vi "Write SerDes GPIO Bank.vi"(0 "gpio bank output":T2, 2 "serdes id":T1=enum."SI 0 Deserializer") -> (4 "serdes id valid":bool)   [LabVIEW 2020, in "GettingStarted_Common_148X_FPGA.lvlib"]
uses:
  GettingStarted_Common_148X_FPGA.lvlib
  <instrlib>/FlexRIO/CSI-2/v2/FPGA/Types/GPIO Bank.ctl
  Types/SerDes Identifier.ctl
  <instrlib>/_niInstr/Basic Elements/v1/FPGA/niInstr Basic Elements v1 FPGA.lvlib
  <vilib>/eio/EIONode/EIONode.xnode
  <vilib>/rvi/eio/common/nirviEmuTemplateMethod_errors.vi
  <instrlib>/FlexRIO/CSI-2/v2/FPGA/NI CSI-2 API FPGA v2.lvlib
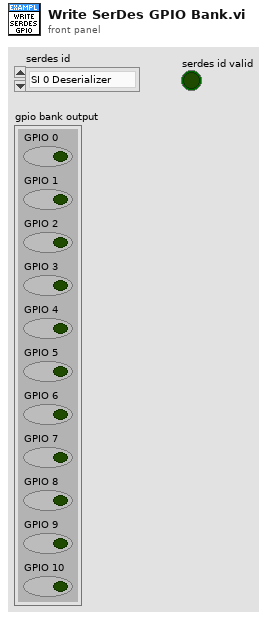
[diagram p1: front panel]
types:
  T1 = typedef "GettingStarted_Common_148X_FPGA.lvlib/SerDes Identifier.ctl" = enum8{"None", "SI 0 Deserializer", "SI 1 Deserializer", "SI 2 Deserializer", "SI 3 Deserializer", "SI 4 Deserializer", "SI 5 Deserializer", "SI 6 Deserializer", "SI 7 Deserializer", "SO 0 Serializer", "SO 1 Serializer", "SO 2 Serializer", "SO 3 Serializer", "SO 4 Serializer", "SO 5 Serializer", "SO 6 Serializer", "SO 7 Serializer", "SI 0 SI 1 Deserializer", "SI 2 SI 3 Deserializer", "SI 4 SI 5 Deserializer", "SI 6 SI 7 Deserializer"}
  T2 = typedef "NI CSI-2 API FPGA v2.lvlib/GPIO Bank.ctl" = cluster{"GPIO 0":bool, "GPIO 1":bool, "GPIO 2":bool, "GPIO 3":bool, "GPIO 4":bool, "GPIO 5":bool, "GPIO 6":bool, "GPIO 7":bool, "GPIO 8":bool, "GPIO 9":bool, "GPIO 10":bool}
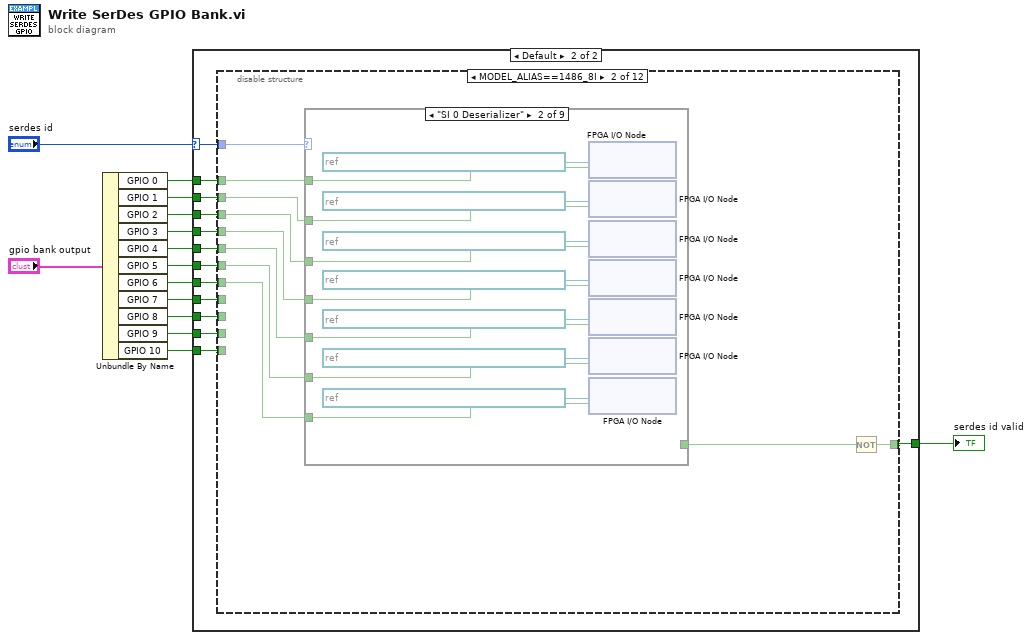
[diagram p0: block diagram]
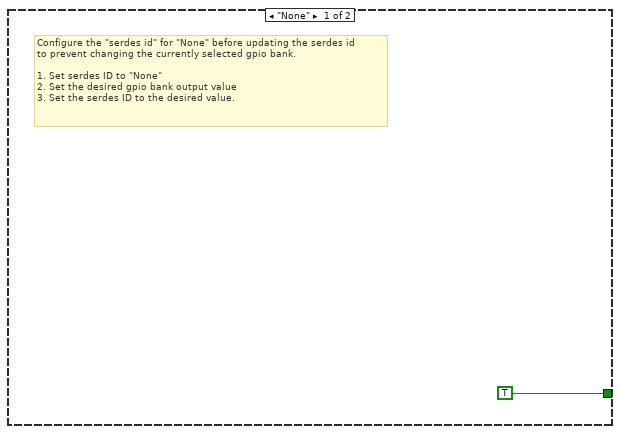
[diagram p2: hidden frame]
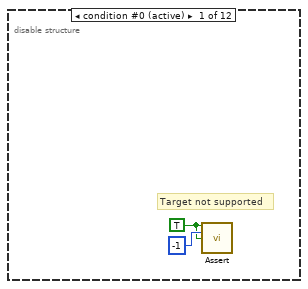
[diagram p3: hidden frame]
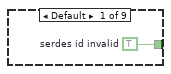
[diagram p4: hidden frame]
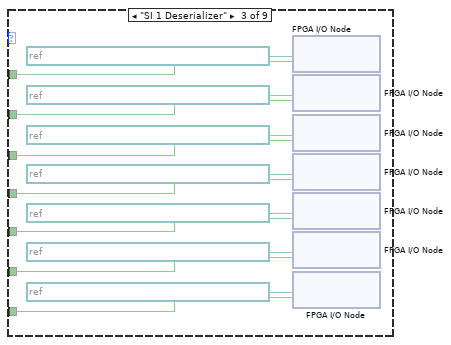
[diagram p5: hidden frame]
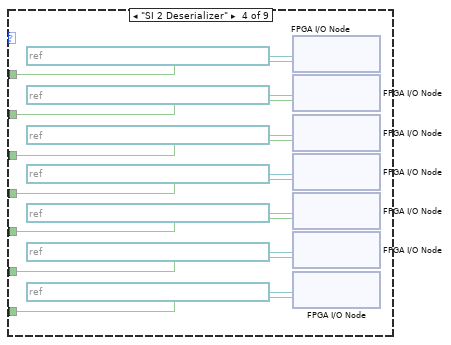
[diagram p6: hidden frame]
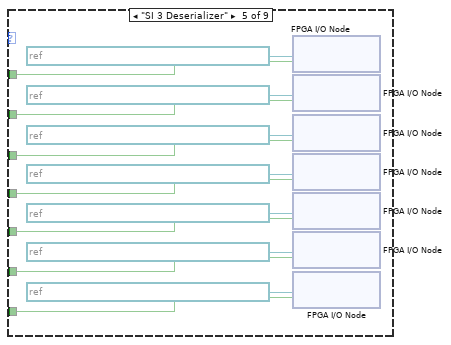
[diagram p7: hidden frame]
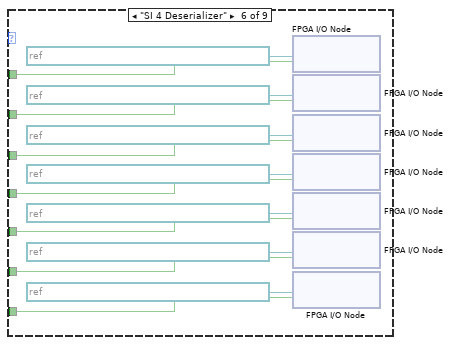
[diagram p8: hidden frame]
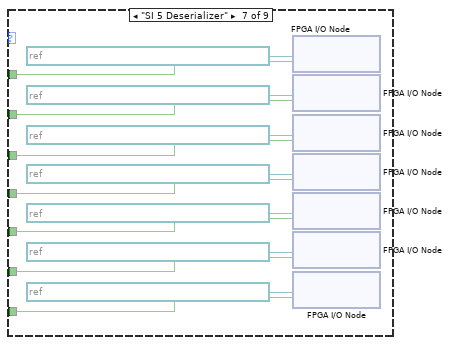
[diagram p9: hidden frame]
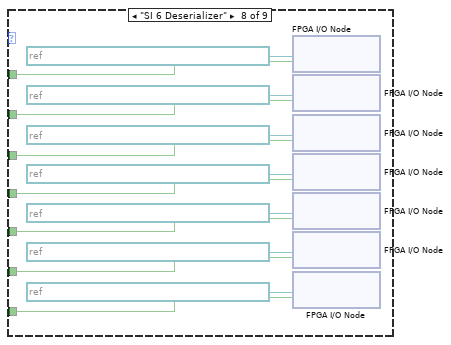
[diagram p10: hidden frame]
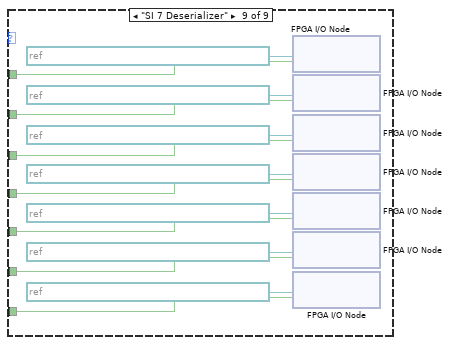
[diagram p11: hidden frame]
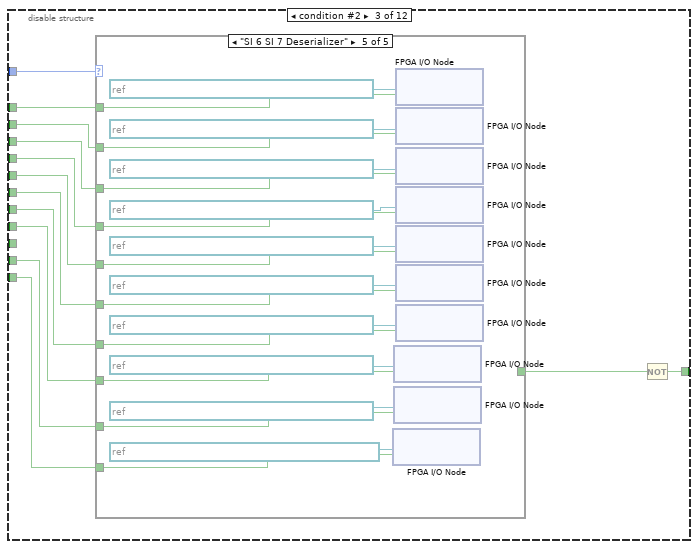
[diagram p12: hidden frame]
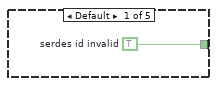
[diagram p13: hidden frame]
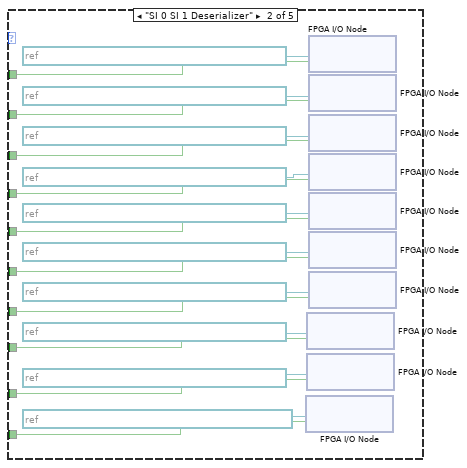
[diagram p14: hidden frame]
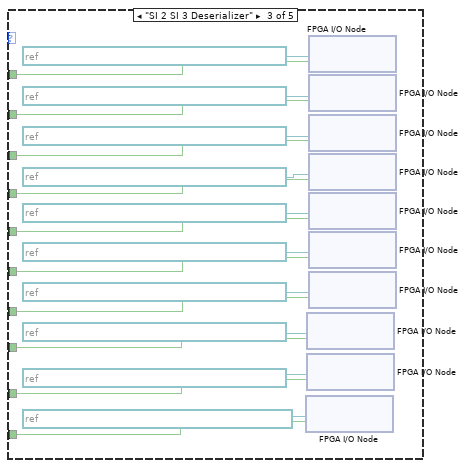
[diagram p15: hidden frame]
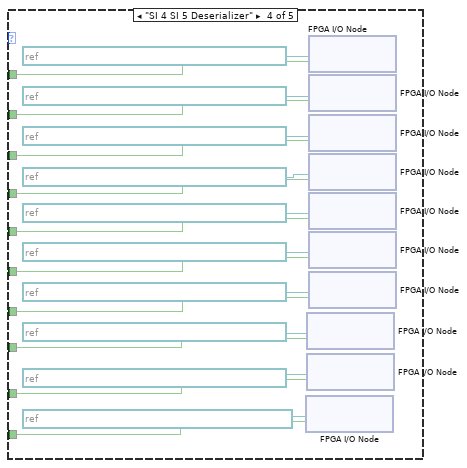
[diagram p16: hidden frame]
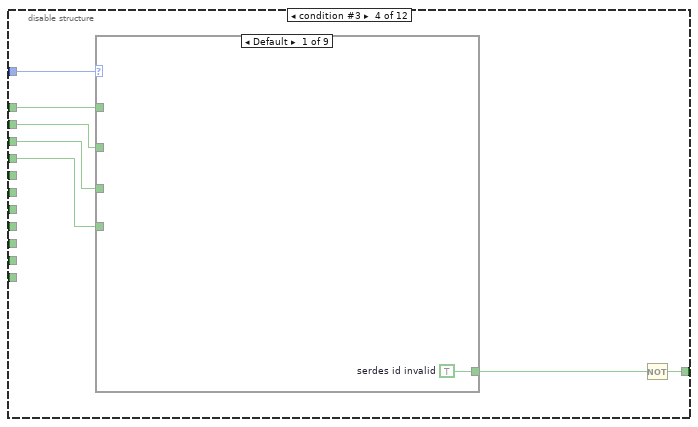
[diagram p17: hidden frame]
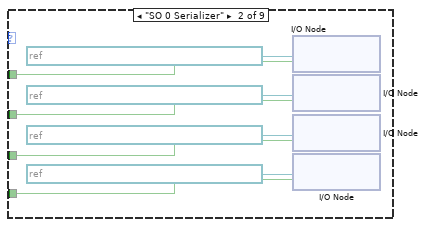
[diagram p18: hidden frame]
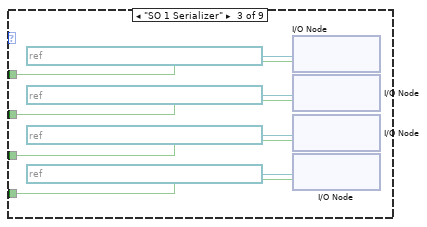
[diagram p19: hidden frame]
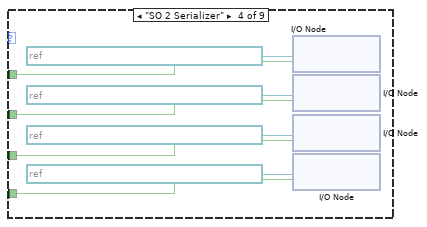
[diagram p20: hidden frame]
diagram:
  n1 = Unbundle By Name("gpio bank output") -> ("GPIO 0"=w13:bool, "GPIO 1"=w12:bool, "GPIO 2"=w11:bool, "GPIO 3"=w10:bool, "GPIO 4"=w9:bool, "GPIO 5"=w8:bool, "GPIO 6"=w7:bool, "GPIO 7"=w6:bool, "GPIO 8"=w5:bool, "GPIO 9"=w4:bool, "GPIO 10"=w3:bool)
  n2 = case shown="Default" "serdes id" {
    selector: "serdes id" -> [_ w16]
    tunnel: w13 -> [_ w28]
    tunnel: w12 -> [_ w27]
    tunnel: w11 -> [_ w26]
    tunnel: w10 -> [_ w25]
    tunnel: w9 -> [_ w24]
    tunnel: w8 -> [_ w23]
    tunnel: w7 -> [_ w22]
    tunnel: w6 -> [_ w21]
    tunnel: w5 -> [_ w20]
    tunnel: w4 -> [_ w19]
    tunnel: w3 -> [_ w18]
    tunnel: [TRUE w17] -> w2
    frame "None" {
      # "Configure the \"serdes id\" for \"None\" before updating the serdes id\nto prevent changing the currently selected gpio bank.\n\n1. Set serdes ID to \"None\" \n2. Set the desired gpio bank output value \n3. Set the serdes ID to the desired value."
    }
    frame Default {
      n3 = disable-structure shown="MODEL_ALIAS==1486_8I" {
        disable-tunnel: w16 -> [_ w40 w166 w254 w329 w431 w558 w645 w691 w797 w860 w995]
        disable-tunnel: w28 -> [_ w39 w165 w253 w328 w430 w557 w644 w690 w796 w859 w994]
        disable-tunnel: w27 -> [_ w38 w164 w252 w327 w429 w556 w643 _ _ w858 w993]
        disable-tunnel: w26 -> [_ w37 w163 w251 w326 w428 w555 w642 _ _ w857 w992]
        disable-tunnel: w25 -> [_ w36 w162 w250 w325 w427 w554 w641 w689 w795 w856 w991]
        disable-tunnel: w24 -> [_ w35 w161 _ w324 w426 w553 w640 w688 w794 w855 w990]
        disable-tunnel: w23 -> [_ w34 w160 _ w323 w425 w552 w639 _ _ w854 w989]
        disable-tunnel: w22 -> [_ w33 w159 _ w322 w424 w551 w638 w687 w793 w853 w988]
        disable-tunnel: w21 -> [_ _ w156 _ _ w421 w548 w635 w684 w790 w850 w985]
        disable-tunnel: w20 -> [_ _ _ _ _ _ w547 w634 w683 w789 w849 w984]
        disable-tunnel: w19 -> [_ _ w155 _ _ w420 w546 w633 _ _ w848 w983]
        disable-tunnel: w18 -> [_ _ w154 _ _ w419 w545 w632 _ _ w847 w982]
        disable-tunnel: [_ w31 w157 w248 w320 w422 w549 w636 w685 w791 w851 w986] -> w17
        frame condition #0 (active) {
          w29 = TRUE ("assert")
          # "Target not supported"
          n4 = call <instrlib>:"Assert.vi"("assert"=w29, "error code"=-1, "enable show error"=w29) -> ()  [unwired: 13 in]
        }
        frame condition #1 {
          n5 = case shown="\"SI 0 Deserializer\"" w40 {
            tunnel: w39 -> [_ w48 w62 w76 w90 w104 w118 w132 w146]
            tunnel: w38 -> [_ w47 w61 w75 w89 w103 w117 w131 w145]
            tunnel: w37 -> [_ w46 w60 w74 w88 w102 w116 w130 w144]
            tunnel: w36 -> [_ w45 w59 w73 w87 w101 w115 w129 w143]
            tunnel: w35 -> [_ w44 w58 w72 w86 w100 w114 w128 w142]
            tunnel: w34 -> [_ w43 w57 w71 w85 w99 w113 w127 w141]
            tunnel: w33 -> [_ w42 w56 w70 w84 w98 w112 w126 w140]
            tunnel: [w41 _ _ _ _ _ _ _ _] -> w32
            frame Default {
              w41 = TRUE  # serdes id invalid
            }
            frame "SI 0 Deserializer" {
              n6 = xnode "FPGA I/O Node"("I/O Item"=w48, "FPGA I/O In"=refnum<k21> "IO Socket\\SI 0 Deserializer GPIO 0 Output") -> ()  [unwired: 1 out]
              n7 = xnode "FPGA I/O Node"("I/O Item"=w47, "FPGA I/O In"=refnum<k21> "IO Socket\\SI 0 Deserializer GPIO 1 Output") -> ()  [unwired: 1 out]
              n8 = xnode "FPGA I/O Node"("I/O Item"=w46, "FPGA I/O In"=refnum<k21> "IO Socket\\SI 0 Deserializer GPIO 2 Output") -> ()  [unwired: 1 out]
              n9 = xnode "FPGA I/O Node"("I/O Item"=w45, "FPGA I/O In"=refnum<k21> "IO Socket\\SI 0 Deserializer GPIO 3 Output") -> ()  [unwired: 1 out]
              n10 = xnode "FPGA I/O Node"("I/O Item"=w44, "FPGA I/O In"=refnum<k21> "IO Socket\\SI 0 Deserializer GPIO 4 Output") -> ()  [unwired: 1 out]
              n11 = xnode "FPGA I/O Node"("I/O Item"=w43, "FPGA I/O In"=refnum<k21> "IO Socket\\SI 0 Deserializer GPIO 5 Output") -> ()  [unwired: 1 out]
              n12 = xnode "FPGA I/O Node"("I/O Item"=w42, "FPGA I/O In"=refnum<k21> "IO Socket\\SI 0 Deserializer GPIO 6 Output") -> ()  [unwired: 1 out]
            }
            frame "SI 1 Deserializer" {
              n13 = xnode "FPGA I/O Node"("I/O Item"=w62, "FPGA I/O In"=refnum<k21> "IO Socket\\SI 1 Deserializer GPIO 0 Output") -> ()  [unwired: 1 out]
              n14 = xnode "FPGA I/O Node"("I/O Item"=w61, "FPGA I/O In"=refnum<k21> "IO Socket\\SI 1 Deserializer GPIO 1 Output") -> ()  [unwired: 1 out]
              n15 = xnode "FPGA I/O Node"("I/O Item"=w60, "FPGA I/O In"=refnum<k21> "IO Socket\\SI 1 Deserializer GPIO 2 Output") -> ()  [unwired: 1 out]
              n16 = xnode "FPGA I/O Node"("I/O Item"=w59, "FPGA I/O In"=refnum<k21> "IO Socket\\SI 1 Deserializer GPIO 3 Output") -> ()  [unwired: 1 out]
              n17 = xnode "FPGA I/O Node"("I/O Item"=w58, "FPGA I/O In"=refnum<k21> "IO Socket\\SI 1 Deserializer GPIO 4 Output") -> ()  [unwired: 1 out]
              n18 = xnode "FPGA I/O Node"("I/O Item"=w57, "FPGA I/O In"=refnum<k21> "IO Socket\\SI 1 Deserializer GPIO 5 Output") -> ()  [unwired: 1 out]
              n19 = xnode "FPGA I/O Node"("I/O Item"=w56, "FPGA I/O In"=refnum<k21> "IO Socket\\SI 1 Deserializer GPIO 6 Output") -> ()  [unwired: 1 out]
            }
            frame "SI 2 Deserializer" {
              n20 = xnode "FPGA I/O Node"("I/O Item"=w76, "FPGA I/O In"=refnum<k21> "IO Socket\\SI 2 Deserializer GPIO 0 Output") -> ()  [unwired: 1 out]
              n21 = xnode "FPGA I/O Node"("I/O Item"=w75, "FPGA I/O In"=refnum<k21> "IO Socket\\SI 2 Deserializer GPIO 1 Output") -> ()  [unwired: 1 out]
              n22 = xnode "FPGA I/O Node"("I/O Item"=w74, "FPGA I/O In"=refnum<k21> "IO Socket\\SI 2 Deserializer GPIO 2 Output") -> ()  [unwired: 1 out]
              n23 = xnode "FPGA I/O Node"("I/O Item"=w73, "FPGA I/O In"=refnum<k21> "IO Socket\\SI 2 Deserializer GPIO 3 Output") -> ()  [unwired: 1 out]
              n24 = xnode "FPGA I/O Node"("I/O Item"=w72, "FPGA I/O In"=refnum<k21> "IO Socket\\SI 2 Deserializer GPIO 4 Output") -> ()  [unwired: 1 out]
              n25 = xnode "FPGA I/O Node"("I/O Item"=w71, "FPGA I/O In"=refnum<k21> "IO Socket\\SI 2 Deserializer GPIO 5 Output") -> ()  [unwired: 1 out]
              n26 = xnode "FPGA I/O Node"("I/O Item"=w70, "FPGA I/O In"=refnum<k21> "IO Socket\\SI 2 Deserializer GPIO 6 Output") -> ()  [unwired: 1 out]
            }
            frame "SI 3 Deserializer" {
              n27 = xnode "FPGA I/O Node"("I/O Item"=w90, "FPGA I/O In"=refnum<k21> "IO Socket\\SI 3 Deserializer GPIO 0 Output") -> ()  [unwired: 1 out]
              n28 = xnode "FPGA I/O Node"("I/O Item"=w89, "FPGA I/O In"=refnum<k21> "IO Socket\\SI 3 Deserializer GPIO 1 Output") -> ()  [unwired: 1 out]
              n29 = xnode "FPGA I/O Node"("I/O Item"=w88, "FPGA I/O In"=refnum<k21> "IO Socket\\SI 3 Deserializer GPIO 2 Output") -> ()  [unwired: 1 out]
              n30 = xnode "FPGA I/O Node"("I/O Item"=w87, "FPGA I/O In"=refnum<k21> "IO Socket\\SI 3 Deserializer GPIO 3 Output") -> ()  [unwired: 1 out]
              n31 = xnode "FPGA I/O Node"("I/O Item"=w86, "FPGA I/O In"=refnum<k21> "IO Socket\\SI 3 Deserializer GPIO 4 Output") -> ()  [unwired: 1 out]
              n32 = xnode "FPGA I/O Node"("I/O Item"=w85, "FPGA I/O In"=refnum<k21> "IO Socket\\SI 3 Deserializer GPIO 5 Output") -> ()  [unwired: 1 out]
              n33 = xnode "FPGA I/O Node"("I/O Item"=w84, "FPGA I/O In"=refnum<k21> "IO Socket\\SI 3 Deserializer GPIO 6 Output") -> ()  [unwired: 1 out]
            }
            frame "SI 4 Deserializer" {
              n34 = xnode "FPGA I/O Node"("I/O Item"=w104, "FPGA I/O In"=refnum<k21> "IO Socket\\SI 4 Deserializer GPIO 0 Output") -> ()  [unwired: 1 out]
              n35 = xnode "FPGA I/O Node"("I/O Item"=w103, "FPGA I/O In"=refnum<k21> "IO Socket\\SI 4 Deserializer GPIO 1 Output") -> ()  [unwired: 1 out]
              n36 = xnode "FPGA I/O Node"("I/O Item"=w102, "FPGA I/O In"=refnum<k21> "IO Socket\\SI 4 Deserializer GPIO 2 Output") -> ()  [unwired: 1 out]
              n37 = xnode "FPGA I/O Node"("I/O Item"=w101, "FPGA I/O In"=refnum<k21> "IO Socket\\SI 4 Deserializer GPIO 3 Output") -> ()  [unwired: 1 out]
              n38 = xnode "FPGA I/O Node"("I/O Item"=w100, "FPGA I/O In"=refnum<k21> "IO Socket\\SI 4 Deserializer GPIO 4 Output") -> ()  [unwired: 1 out]
              n39 = xnode "FPGA I/O Node"("I/O Item"=w99, "FPGA I/O In"=refnum<k21> "IO Socket\\SI 4 Deserializer GPIO 5 Output") -> ()  [unwired: 1 out]
              n40 = xnode "FPGA I/O Node"("I/O Item"=w98, "FPGA I/O In"=refnum<k21> "IO Socket\\SI 4 Deserializer GPIO 6 Output") -> ()  [unwired: 1 out]
            }
            frame "SI 5 Deserializer" {
              n41 = xnode "FPGA I/O Node"("I/O Item"=w118, "FPGA I/O In"=refnum<k21> "IO Socket\\SI 5 Deserializer GPIO 0 Output") -> ()  [unwired: 1 out]
              n42 = xnode "FPGA I/O Node"("I/O Item"=w117, "FPGA I/O In"=refnum<k21> "IO Socket\\SI 5 Deserializer GPIO 1 Output") -> ()  [unwired: 1 out]
              n43 = xnode "FPGA I/O Node"("I/O Item"=w116, "FPGA I/O In"=refnum<k21> "IO Socket\\SI 5 Deserializer GPIO 2 Output") -> ()  [unwired: 1 out]
              n44 = xnode "FPGA I/O Node"("I/O Item"=w115, "FPGA I/O In"=refnum<k21> "IO Socket\\SI 5 Deserializer GPIO 3 Output") -> ()  [unwired: 1 out]
              n45 = xnode "FPGA I/O Node"("I/O Item"=w114, "FPGA I/O In"=refnum<k21> "IO Socket\\SI 5 Deserializer GPIO 4 Output") -> ()  [unwired: 1 out]
              n46 = xnode "FPGA I/O Node"("I/O Item"=w113, "FPGA I/O In"=refnum<k21> "IO Socket\\SI 5 Deserializer GPIO 5 Output") -> ()  [unwired: 1 out]
              n47 = xnode "FPGA I/O Node"("I/O Item"=w112, "FPGA I/O In"=refnum<k21> "IO Socket\\SI 5 Deserializer GPIO 6 Output") -> ()  [unwired: 1 out]
            }
            frame "SI 6 Deserializer" {
              n48 = xnode "FPGA I/O Node"("I/O Item"=w132, "FPGA I/O In"=refnum<k21> "IO Socket\\SI 6 Deserializer GPIO 0 Output") -> ()  [unwired: 1 out]
              n49 = xnode "FPGA I/O Node"("I/O Item"=w131, "FPGA I/O In"=refnum<k21> "IO Socket\\SI 6 Deserializer GPIO 1 Output") -> ()  [unwired: 1 out]
              n50 = xnode "FPGA I/O Node"("I/O Item"=w130, "FPGA I/O In"=refnum<k21> "IO Socket\\SI 6 Deserializer GPIO 2 Output") -> ()  [unwired: 1 out]
              n51 = xnode "FPGA I/O Node"("I/O Item"=w129, "FPGA I/O In"=refnum<k21> "IO Socket\\SI 6 Deserializer GPIO 3 Output") -> ()  [unwired: 1 out]
              n52 = xnode "FPGA I/O Node"("I/O Item"=w128, "FPGA I/O In"=refnum<k21> "IO Socket\\SI 6 Deserializer GPIO 4 Output") -> ()  [unwired: 1 out]
              n53 = xnode "FPGA I/O Node"("I/O Item"=w127, "FPGA I/O In"=refnum<k21> "IO Socket\\SI 6 Deserializer GPIO 5 Output") -> ()  [unwired: 1 out]
              n54 = xnode "FPGA I/O Node"("I/O Item"=w126, "FPGA I/O In"=refnum<k21> "IO Socket\\SI 6 Deserializer GPIO 6 Output") -> ()  [unwired: 1 out]
            }
            frame "SI 7 Deserializer" {
              n55 = xnode "FPGA I/O Node"("I/O Item"=w146, "FPGA I/O In"=refnum<k21> "IO Socket\\SI 7 Deserializer GPIO 0 Output") -> ()  [unwired: 1 out]
              n56 = xnode "FPGA I/O Node"("I/O Item"=w145, "FPGA I/O In"=refnum<k21> "IO Socket\\SI 7 Deserializer GPIO 1 Output") -> ()  [unwired: 1 out]
              n57 = xnode "FPGA I/O Node"("I/O Item"=w144, "FPGA I/O In"=refnum<k21> "IO Socket\\SI 7 Deserializer GPIO 2 Output") -> ()  [unwired: 1 out]
              n58 = xnode "FPGA I/O Node"("I/O Item"=w143, "FPGA I/O In"=refnum<k21> "IO Socket\\SI 7 Deserializer GPIO 3 Output") -> ()  [unwired: 1 out]
              n59 = xnode "FPGA I/O Node"("I/O Item"=w142, "FPGA I/O In"=refnum<k21> "IO Socket\\SI 7 Deserializer GPIO 4 Output") -> ()  [unwired: 1 out]
              n60 = xnode "FPGA I/O Node"("I/O Item"=w141, "FPGA I/O In"=refnum<k21> "IO Socket\\SI 7 Deserializer GPIO 5 Output") -> ()  [unwired: 1 out]
              n61 = xnode "FPGA I/O Node"("I/O Item"=w140, "FPGA I/O In"=refnum<k21> "IO Socket\\SI 7 Deserializer GPIO 6 Output") -> ()  [unwired: 1 out]
            }
          }
          n62 = Not(x=w32) -> (.not. x?=w31:bool)
        }
        frame condition #2 {
          n63 = case shown="\"SI 6 SI 7 Deserializer\"" w166 {
            tunnel: w165 -> [_ w187 w207 w227 w247]
            tunnel: w164 -> [_ w186 w206 w226 w246]
            tunnel: w163 -> [_ w185 w205 w225 w245]
            tunnel: w162 -> [_ w184 w204 w224 w244]
            tunnel: w161 -> [_ w183 w203 w223 w243]
            tunnel: w160 -> [_ w182 w202 w222 w242]
            tunnel: w159 -> [_ w181 w201 w221 w241]
            tunnel: [w167 _ _ _ _] -> w158
            tunnel: w156 -> [_ w170 w190 w210 w230]
            tunnel: w155 -> [_ w169 w189 w209 w229]
            tunnel: w154 -> [_ w168 w188 w208 w228]
            frame Default {
              w167 = TRUE  # serdes id invalid
            }
            frame "SI 0 SI 1 Deserializer" {
              n64 = xnode "FPGA I/O Node"("I/O Item"=w168, "FPGA I/O In"=refnum<k21> "IO Socket\\SI 0 SI 1 Deserializer GPIO 10 Output") -> ()  [unwired: 1 out]
              n65 = xnode "FPGA I/O Node"("I/O Item"=w170, "FPGA I/O In"=refnum<k21> "IO Socket\\SI 0 SI 1 Deserializer GPIO 7 Output") -> ()  [unwired: 1 out]
              n66 = xnode "FPGA I/O Node"("I/O Item"=w169, "FPGA I/O In"=refnum<k21> "IO Socket\\SI 0 SI 1 Deserializer GPIO 9 Output") -> ()  [unwired: 1 out]
              n67 = xnode "FPGA I/O Node"("I/O Item"=w187, "FPGA I/O In"=refnum<k21> "IO Socket\\SI 0 SI 1 Deserializer GPIO 0 Output") -> ()  [unwired: 1 out]
              n68 = xnode "FPGA I/O Node"("I/O Item"=w186, "FPGA I/O In"=refnum<k21> "IO Socket\\SI 0 SI 1 Deserializer GPIO 1 Output") -> ()  [unwired: 1 out]
              n69 = xnode "FPGA I/O Node"("I/O Item"=w185, "FPGA I/O In"=refnum<k21> "IO Socket\\SI 0 SI 1 Deserializer GPIO 2 Output") -> ()  [unwired: 1 out]
              n70 = xnode "FPGA I/O Node"("I/O Item"=w184, "FPGA I/O In"=refnum<k21> "IO Socket\\SI 0 SI 1 Deserializer GPIO 3 Output") -> ()  [unwired: 1 out]
              n71 = xnode "FPGA I/O Node"("I/O Item"=w183, "FPGA I/O In"=refnum<k21> "IO Socket\\SI 0 SI 1 Deserializer GPIO 4 Output") -> ()  [unwired: 1 out]
              n72 = xnode "FPGA I/O Node"("I/O Item"=w182, "FPGA I/O In"=refnum<k21> "IO Socket\\SI 0 SI 1 Deserializer GPIO 5 Output") -> ()  [unwired: 1 out]
              n73 = xnode "FPGA I/O Node"("I/O Item"=w181, "FPGA I/O In"=refnum<k21> "IO Socket\\SI 0 SI 1 Deserializer GPIO 6 Output") -> ()  [unwired: 1 out]
            }
            frame "SI 2 SI 3 Deserializer" {
              n74 = xnode "FPGA I/O Node"("I/O Item"=w188, "FPGA I/O In"=refnum<k21> "IO Socket\\SI 2 SI 3 Deserializer GPIO 10 Output") -> ()  [unwired: 1 out]
              n75 = xnode "FPGA I/O Node"("I/O Item"=w190, "FPGA I/O In"=refnum<k21> "IO Socket\\SI 2 SI 3 Deserializer GPIO 7 Output") -> ()  [unwired: 1 out]
              n76 = xnode "FPGA I/O Node"("I/O Item"=w189, "FPGA I/O In"=refnum<k21> "IO Socket\\SI 2 SI 3 Deserializer GPIO 9 Output") -> ()  [unwired: 1 out]
              n77 = xnode "FPGA I/O Node"("I/O Item"=w207, "FPGA I/O In"=refnum<k21> "IO Socket\\SI 2 SI 3 Deserializer GPIO 0 Output") -> ()  [unwired: 1 out]
              n78 = xnode "FPGA I/O Node"("I/O Item"=w206, "FPGA I/O In"=refnum<k21> "IO Socket\\SI 2 SI 3 Deserializer GPIO 1 Output") -> ()  [unwired: 1 out]
              n79 = xnode "FPGA I/O Node"("I/O Item"=w205, "FPGA I/O In"=refnum<k21> "IO Socket\\SI 2 SI 3 Deserializer GPIO 2 Output") -> ()  [unwired: 1 out]
              n80 = xnode "FPGA I/O Node"("I/O Item"=w204, "FPGA I/O In"=refnum<k21> "IO Socket\\SI 2 SI 3 Deserializer GPIO 3 Output") -> ()  [unwired: 1 out]
              n81 = xnode "FPGA I/O Node"("I/O Item"=w203, "FPGA I/O In"=refnum<k21> "IO Socket\\SI 2 SI 3 Deserializer GPIO 4 Output") -> ()  [unwired: 1 out]
              n82 = xnode "FPGA I/O Node"("I/O Item"=w202, "FPGA I/O In"=refnum<k21> "IO Socket\\SI 2 SI 3 Deserializer GPIO 5 Output") -> ()  [unwired: 1 out]
              n83 = xnode "FPGA I/O Node"("I/O Item"=w201, "FPGA I/O In"=refnum<k21> "IO Socket\\SI 2 SI 3 Deserializer GPIO 6 Output") -> ()  [unwired: 1 out]
            }
            frame "SI 4 SI 5 Deserializer" {
              n84 = xnode "FPGA I/O Node"("I/O Item"=w208, "FPGA I/O In"=refnum<k21> "IO Socket\\SI 4 SI 5 Deserializer GPIO 10 Output") -> ()  [unwired: 1 out]
              n85 = xnode "FPGA I/O Node"("I/O Item"=w210, "FPGA I/O In"=refnum<k21> "IO Socket\\SI 4 SI 5 Deserializer GPIO 7 Output") -> ()  [unwired: 1 out]
              n86 = xnode "FPGA I/O Node"("I/O Item"=w209, "FPGA I/O In"=refnum<k21> "IO Socket\\SI 4 SI 5 Deserializer GPIO 9 Output") -> ()  [unwired: 1 out]
              n87 = xnode "FPGA I/O Node"("I/O Item"=w227, "FPGA I/O In"=refnum<k21> "IO Socket\\SI 4 SI 5 Deserializer GPIO 0 Output") -> ()  [unwired: 1 out]
              n88 = xnode "FPGA I/O Node"("I/O Item"=w226, "FPGA I/O In"=refnum<k21> "IO Socket\\SI 4 SI 5 Deserializer GPIO 1 Output") -> ()  [unwired: 1 out]
              n89 = xnode "FPGA I/O Node"("I/O Item"=w225, "FPGA I/O In"=refnum<k21> "IO Socket\\SI 4 SI 5 Deserializer GPIO 2 Output") -> ()  [unwired: 1 out]
              n90 = xnode "FPGA I/O Node"("I/O Item"=w224, "FPGA I/O In"=refnum<k21> "IO Socket\\SI 4 SI 5 Deserializer GPIO 3 Output") -> ()  [unwired: 1 out]
              n91 = xnode "FPGA I/O Node"("I/O Item"=w223, "FPGA I/O In"=refnum<k21> "IO Socket\\SI 4 SI 5 Deserializer GPIO 4 Output") -> ()  [unwired: 1 out]
              n92 = xnode "FPGA I/O Node"("I/O Item"=w222, "FPGA I/O In"=refnum<k21> "IO Socket\\SI 4 SI 5 Deserializer GPIO 5 Output") -> ()  [unwired: 1 out]
              n93 = xnode "FPGA I/O Node"("I/O Item"=w221, "FPGA I/O In"=refnum<k21> "IO Socket\\SI 4 SI 5 Deserializer GPIO 6 Output") -> ()  [unwired: 1 out]
            }
            frame "SI 6 SI 7 Deserializer" {
              n94 = xnode "FPGA I/O Node"("I/O Item"=w228, "FPGA I/O In"=refnum<k21> "IO Socket\\SI 6 SI 7 Deserializer GPIO 10 Output") -> ()  [unwired: 1 out]
              n95 = xnode "FPGA I/O Node"("I/O Item"=w230, "FPGA I/O In"=refnum<k21> "IO Socket\\SI 6 SI 7 Deserializer GPIO 7 Output") -> ()  [unwired: 1 out]
              n96 = xnode "FPGA I/O Node"("I/O Item"=w229, "FPGA I/O In"=refnum<k21> "IO Socket\\SI 6 SI 7 Deserializer GPIO 9 Output") -> ()  [unwired: 1 out]
              n97 = xnode "FPGA I/O Node"("I/O Item"=w247, "FPGA I/O In"=refnum<k21> "IO Socket\\SI 6 SI 7 Deserializer GPIO 0 Output") -> ()  [unwired: 1 out]
              n98 = xnode "FPGA I/O Node"("I/O Item"=w246, "FPGA I/O In"=refnum<k21> "IO Socket\\SI 6 SI 7 Deserializer GPIO 1 Output") -> ()  [unwired: 1 out]
              n99 = xnode "FPGA I/O Node"("I/O Item"=w245, "FPGA I/O In"=refnum<k21> "IO Socket\\SI 6 SI 7 Deserializer GPIO 2 Output") -> ()  [unwired: 1 out]
              n100 = xnode "FPGA I/O Node"("I/O Item"=w244, "FPGA I/O In"=refnum<k21> "IO Socket\\SI 6 SI 7 Deserializer GPIO 3 Output") -> ()  [unwired: 1 out]
              n101 = xnode "FPGA I/O Node"("I/O Item"=w243, "FPGA I/O In"=refnum<k21> "IO Socket\\SI 6 SI 7 Deserializer GPIO 4 Output") -> ()  [unwired: 1 out]
              n102 = xnode "FPGA I/O Node"("I/O Item"=w242, "FPGA I/O In"=refnum<k21> "IO Socket\\SI 6 SI 7 Deserializer GPIO 5 Output") -> ()  [unwired: 1 out]
              n103 = xnode "FPGA I/O Node"("I/O Item"=w241, "FPGA I/O In"=refnum<k21> "IO Socket\\SI 6 SI 7 Deserializer GPIO 6 Output") -> ()  [unwired: 1 out]
            }
          }
          n104 = Not(x=w158) -> (.not. x?=w157:bool)
        }
        frame condition #3 {
          n105 = case shown="Default" w254 {
            tunnel: w253 -> [_ w259 w267 w275 w283 w291 w299 w307 w315]
            tunnel: w252 -> [_ w258 w266 w274 w282 w290 w298 w306 w314]
            tunnel: w251 -> [_ w257 w265 w273 w281 w289 w297 w305 w313]
            tunnel: w250 -> [_ w256 w264 w272 w280 w288 w296 w304 w312]
            tunnel: [w255 _ _ _ _ _ _ _ _] -> w249
            frame Default {
              w255 = TRUE  # serdes id invalid
            }
            frame "SO 0 Serializer" {
              n106 = xnode "I/O Node"("I/O Item"=w259, "FPGA I/O In"=refnum<k21> "IO Socket\\SO 0 Serializer GPIO 0 Output") -> ()  [unwired: 1 out]
              n107 = xnode "I/O Node"("I/O Item"=w258, "FPGA I/O In"=refnum<k21> "IO Socket\\SO 0 Serializer GPIO 1 Output") -> ()  [unwired: 1 out]
              n108 = xnode "I/O Node"("I/O Item"=w257, "FPGA I/O In"=refnum<k21> "IO Socket\\SO 0 Serializer GPIO 2 Output") -> ()  [unwired: 1 out]
              n109 = xnode "I/O Node"("I/O Item"=w256, "FPGA I/O In"=refnum<k21> "IO Socket\\SO 0 Serializer GPIO 3 Output") -> ()  [unwired: 1 out]
            }
            frame "SO 1 Serializer" {
              n110 = xnode "I/O Node"("I/O Item"=w267, "FPGA I/O In"=refnum<k21> "IO Socket\\SO 1 Serializer GPIO 0 Output") -> ()  [unwired: 1 out]
              n111 = xnode "I/O Node"("I/O Item"=w266, "FPGA I/O In"=refnum<k21> "IO Socket\\SO 1 Serializer GPIO 1 Output") -> ()  [unwired: 1 out]
              n112 = xnode "I/O Node"("I/O Item"=w265, "FPGA I/O In"=refnum<k21> "IO Socket\\SO 1 Serializer GPIO 2 Output") -> ()  [unwired: 1 out]
              n113 = xnode "I/O Node"("I/O Item"=w264, "FPGA I/O In"=refnum<k21> "IO Socket\\SO 1 Serializer GPIO 3 Output") -> ()  [unwired: 1 out]
            }
            frame "SO 2 Serializer" {
              n114 = xnode "I/O Node"("I/O Item"=w275, "FPGA I/O In"=refnum<k21> "IO Socket\\SO 2 Serializer GPIO 0 Output") -> ()  [unwired: 1 out]
              n115 = xnode "I/O Node"("I/O Item"=w274, "FPGA I/O In"=refnum<k21> "IO Socket\\SO 2 Serializer GPIO 1 Output") -> ()  [unwired: 1 out]
              n116 = xnode "I/O Node"("I/O Item"=w273, "FPGA I/O In"=refnum<k21> "IO Socket\\SO 2 Serializer GPIO 2 Output") -> ()  [unwired: 1 out]
              n117 = xnode "I/O Node"("I/O Item"=w272, "FPGA I/O In"=refnum<k21> "IO Socket\\SO 2 Serializer GPIO 3 Output") -> ()  [unwired: 1 out]
            }
            frame "SO 3 Serializer" {
              n118 = xnode "I/O Node"("I/O Item"=w283, "FPGA I/O In"=refnum<k21> "IO Socket\\SO 3 Serializer GPIO 0 Output") -> ()  [unwired: 1 out]
              n119 = xnode "I/O Node"("I/O Item"=w282, "FPGA I/O In"=refnum<k21> "IO Socket\\SO 3 Serializer GPIO 1 Output") -> ()  [unwired: 1 out]
              n120 = xnode "I/O Node"("I/O Item"=w281, "FPGA I/O In"=refnum<k21> "IO Socket\\SO 3 Serializer GPIO 2 Output") -> ()  [unwired: 1 out]
              n121 = xnode "I/O Node"("I/O Item"=w280, "FPGA I/O In"=refnum<k21> "IO Socket\\SO 3 Serializer GPIO 3 Output") -> ()  [unwired: 1 out]
            }
            frame "SO 4 Serializer" {
              n122 = xnode "I/O Node"("I/O Item"=w291, "FPGA I/O In"=refnum<k21> "IO Socket\\SO 4 Serializer GPIO 0 Output") -> ()  [unwired: 1 out]
              n123 = xnode "I/O Node"("I/O Item"=w290, "FPGA I/O In"=refnum<k21> "IO Socket\\SO 4 Serializer GPIO 1 Output") -> ()  [unwired: 1 out]
              n124 = xnode "I/O Node"("I/O Item"=w289, "FPGA I/O In"=refnum<k21> "IO Socket\\SO 4 Serializer GPIO 2 Output") -> ()  [unwired: 1 out]
              n125 = xnode "I/O Node"("I/O Item"=w288, "FPGA I/O In"=refnum<k21> "IO Socket\\SO 4 Serializer GPIO 3 Output") -> ()  [unwired: 1 out]
            }
            frame "SO 5 Serializer" {
              n126 = xnode "I/O Node"("I/O Item"=w299, "FPGA I/O In"=refnum<k21> "IO Socket\\SO 5 Serializer GPIO 0 Output") -> ()  [unwired: 1 out]
              n127 = xnode "I/O Node"("I/O Item"=w298, "FPGA I/O In"=refnum<k21> "IO Socket\\SO 5 Serializer GPIO 1 Output") -> ()  [unwired: 1 out]
              n128 = xnode "I/O Node"("I/O Item"=w297, "FPGA I/O In"=refnum<k21> "IO Socket\\SO 5 Serializer GPIO 2 Output") -> ()  [unwired: 1 out]
              n129 = xnode "I/O Node"("I/O Item"=w296, "FPGA I/O In"=refnum<k21> "IO Socket\\SO 5 Serializer GPIO 3 Output") -> ()  [unwired: 1 out]
            }
            frame "SO 6 Serializer" {
              n130 = xnode "I/O Node"("I/O Item"=w307, "FPGA I/O In"=refnum<k21> "IO Socket\\SO 6 Serializer GPIO 0 Output") -> ()  [unwired: 1 out]
              n131 = xnode "I/O Node"("I/O Item"=w306, "FPGA I/O In"=refnum<k21> "IO Socket\\SO 6 Serializer GPIO 1 Output") -> ()  [unwired: 1 out]
              n132 = xnode "I/O Node"("I/O Item"=w305, "FPGA I/O In"=refnum<k21> "IO Socket\\SO 6 Serializer GPIO 2 Output") -> ()  [unwired: 1 out]
              n133 = xnode "I/O Node"("I/O Item"=w304, "FPGA I/O In"=refnum<k21> "IO Socket\\SO 6 Serializer GPIO 3 Output") -> ()  [unwired: 1 out]
            }
            frame "SO 7 Serializer" {
              n134 = xnode "I/O Node"("I/O Item"=w315, "FPGA I/O In"=refnum<k21> "IO Socket\\SO 7 Serializer GPIO 0 Output") -> ()  [unwired: 1 out]
              n135 = xnode "I/O Node"("I/O Item"=w314, "FPGA I/O In"=refnum<k21> "IO Socket\\SO 7 Serializer GPIO 1 Output") -> ()  [unwired: 1 out]
              n136 = xnode "I/O Node"("I/O Item"=w313, "FPGA I/O In"=refnum<k21> "IO Socket\\SO 7 Serializer GPIO 2 Output") -> ()  [unwired: 1 out]
              n137 = xnode "I/O Node"("I/O Item"=w312, "FPGA I/O In"=refnum<k21> "IO Socket\\SO 7 Serializer GPIO 3 Output") -> ()  [unwired: 1 out]
            }
          }
          n138 = Not(x=w249) -> (.not. x?=w248:bool)
        }
        frame condition #4 {
          n139 = case shown="\"SI 0 Deserializer\"" w329 {
            tunnel: w328 -> [_ w337 w351 w365 w379 w390 w398 w406 w414]
            tunnel: w327 -> [_ w336 w350 w364 w378 w389 w397 w405 w413]
            tunnel: w326 -> [_ w335 w349 w363 w377 w388 w396 w404 w412]
            tunnel: w325 -> [_ w334 w348 w362 w376 w387 w395 w403 w411]
            tunnel: w324 -> [_ w333 w347 w361 w375 _ _ _ _]
            tunnel: w323 -> [_ w332 w346 w360 w374 _ _ _ _]
            tunnel: w322 -> [_ w331 w345 w359 w373 _ _ _ _]
            tunnel: [w330 _ _ _ _ _ _ _ _] -> w321
            frame Default {
              w330 = TRUE  # serdes id invalid
            }
            frame "SI 0 Deserializer" {
              n140 = xnode "FPGA I/O Node"("I/O Item"=w337, "FPGA I/O In"=refnum<k21> "IO Socket\\SI 0 Deserializer GPIO 0 Output") -> ()  [unwired: 1 out]
              n141 = xnode "FPGA I/O Node"("I/O Item"=w336, "FPGA I/O In"=refnum<k21> "IO Socket\\SI 0 Deserializer GPIO 1 Output") -> ()  [unwired: 1 out]
              n142 = xnode "FPGA I/O Node"("I/O Item"=w335, "FPGA I/O In"=refnum<k21> "IO Socket\\SI 0 Deserializer GPIO 2 Output") -> ()  [unwired: 1 out]
              n143 = xnode "FPGA I/O Node"("I/O Item"=w334, "FPGA I/O In"=refnum<k21> "IO Socket\\SI 0 Deserializer GPIO 3 Output") -> ()  [unwired: 1 out]
              n144 = xnode "FPGA I/O Node"("I/O Item"=w333, "FPGA I/O In"=refnum<k21> "IO Socket\\SI 0 Deserializer GPIO 4 Output") -> ()  [unwired: 1 out]
              n145 = xnode "FPGA I/O Node"("I/O Item"=w332, "FPGA I/O In"=refnum<k21> "IO Socket\\SI 0 Deserializer GPIO 5 Output") -> ()  [unwired: 1 out]
              n146 = xnode "FPGA I/O Node"("I/O Item"=w331, "FPGA I/O In"=refnum<k21> "IO Socket\\SI 0 Deserializer GPIO 6 Output") -> ()  [unwired: 1 out]
            }
            frame "SI 1 Deserializer" {
              n147 = xnode "FPGA I/O Node"("I/O Item"=w351, "FPGA I/O In"=refnum<k21> "IO Socket\\SI 1 Deserializer GPIO 0 Output") -> ()  [unwired: 1 out]
              n148 = xnode "FPGA I/O Node"("I/O Item"=w350, "FPGA I/O In"=refnum<k21> "IO Socket\\SI 1 Deserializer GPIO 1 Output") -> ()  [unwired: 1 out]
              n149 = xnode "FPGA I/O Node"("I/O Item"=w349, "FPGA I/O In"=refnum<k21> "IO Socket\\SI 1 Deserializer GPIO 2 Output") -> ()  [unwired: 1 out]
              n150 = xnode "FPGA I/O Node"("I/O Item"=w348, "FPGA I/O In"=refnum<k21> "IO Socket\\SI 1 Deserializer GPIO 3 Output") -> ()  [unwired: 1 out]
              n151 = xnode "FPGA I/O Node"("I/O Item"=w347, "FPGA I/O In"=refnum<k21> "IO Socket\\SI 1 Deserializer GPIO 4 Output") -> ()  [unwired: 1 out]
              n152 = xnode "FPGA I/O Node"("I/O Item"=w346, "FPGA I/O In"=refnum<k21> "IO Socket\\SI 1 Deserializer GPIO 5 Output") -> ()  [unwired: 1 out]
              n153 = xnode "FPGA I/O Node"("I/O Item"=w345, "FPGA I/O In"=refnum<k21> "IO Socket\\SI 1 Deserializer GPIO 6 Output") -> ()  [unwired: 1 out]
            }
            frame "SI 2 Deserializer" {
              n154 = xnode "FPGA I/O Node"("I/O Item"=w365, "FPGA I/O In"=refnum<k21> "IO Socket\\SI 2 Deserializer GPIO 0 Output") -> ()  [unwired: 1 out]
              n155 = xnode "FPGA I/O Node"("I/O Item"=w364, "FPGA I/O In"=refnum<k21> "IO Socket\\SI 2 Deserializer GPIO 1 Output") -> ()  [unwired: 1 out]
              n156 = xnode "FPGA I/O Node"("I/O Item"=w363, "FPGA I/O In"=refnum<k21> "IO Socket\\SI 2 Deserializer GPIO 2 Output") -> ()  [unwired: 1 out]
              n157 = xnode "FPGA I/O Node"("I/O Item"=w362, "FPGA I/O In"=refnum<k21> "IO Socket\\SI 2 Deserializer GPIO 3 Output") -> ()  [unwired: 1 out]
              n158 = xnode "FPGA I/O Node"("I/O Item"=w361, "FPGA I/O In"=refnum<k21> "IO Socket\\SI 2 Deserializer GPIO 4 Output") -> ()  [unwired: 1 out]
              n159 = xnode "FPGA I/O Node"("I/O Item"=w360, "FPGA I/O In"=refnum<k21> "IO Socket\\SI 2 Deserializer GPIO 5 Output") -> ()  [unwired: 1 out]
              n160 = xnode "FPGA I/O Node"("I/O Item"=w359, "FPGA I/O In"=refnum<k21> "IO Socket\\SI 2 Deserializer GPIO 6 Output") -> ()  [unwired: 1 out]
            }
            frame "SI 3 Deserializer" {
              n161 = xnode "FPGA I/O Node"("I/O Item"=w379, "FPGA I/O In"=refnum<k21> "IO Socket\\SI 3 Deserializer GPIO 0 Output") -> ()  [unwired: 1 out]
              n162 = xnode "FPGA I/O Node"("I/O Item"=w378, "FPGA I/O In"=refnum<k21> "IO Socket\\SI 3 Deserializer GPIO 1 Output") -> ()  [unwired: 1 out]
              n163 = xnode "FPGA I/O Node"("I/O Item"=w377, "FPGA I/O In"=refnum<k21> "IO Socket\\SI 3 Deserializer GPIO 2 Output") -> ()  [unwired: 1 out]
              n164 = xnode "FPGA I/O Node"("I/O Item"=w376, "FPGA I/O In"=refnum<k21> "IO Socket\\SI 3 Deserializer GPIO 3 Output") -> ()  [unwired: 1 out]
              n165 = xnode "FPGA I/O Node"("I/O Item"=w375, "FPGA I/O In"=refnum<k21> "IO Socket\\SI 3 Deserializer GPIO 4 Output") -> ()  [unwired: 1 out]
              n166 = xnode "FPGA I/O Node"("I/O Item"=w374, "FPGA I/O In"=refnum<k21> "IO Socket\\SI 3 Deserializer GPIO 5 Output") -> ()  [unwired: 1 out]
              n167 = xnode "FPGA I/O Node"("I/O Item"=w373, "FPGA I/O In"=refnum<k21> "IO Socket\\SI 3 Deserializer GPIO 6 Output") -> ()  [unwired: 1 out]
            }
            frame "SO 0 Serializer" {
              n168 = xnode "FPGA I/O Node"("I/O Item"=w390, "FPGA I/O In"=refnum<k21> "IO Socket\\SO 0 Serializer GPIO 0 Output") -> ()  [unwired: 1 out]
              n169 = xnode "FPGA I/O Node"("I/O Item"=w389, "FPGA I/O In"=refnum<k21> "IO Socket\\SO 0 Serializer GPIO 1 Output") -> ()  [unwired: 1 out]
              n170 = xnode "FPGA I/O Node"("I/O Item"=w388, "FPGA I/O In"=refnum<k21> "IO Socket\\SO 0 Serializer GPIO 2 Output") -> ()  [unwired: 1 out]
              n171 = xnode "FPGA I/O Node"("I/O Item"=w387, "FPGA I/O In"=refnum<k21> "IO Socket\\SO 0 Serializer GPIO 3 Output") -> ()  [unwired: 1 out]
            }
            frame "SO 1 Serializer" {
              n172 = xnode "FPGA I/O Node"("I/O Item"=w398, "FPGA I/O In"=refnum<k21> "IO Socket\\SO 1 Serializer GPIO 0 Output") -> ()  [unwired: 1 out]
              n173 = xnode "FPGA I/O Node"("I/O Item"=w397, "FPGA I/O In"=refnum<k21> "IO Socket\\SO 1 Serializer GPIO 1 Output") -> ()  [unwired: 1 out]
              n174 = xnode "FPGA I/O Node"("I/O Item"=w396, "FPGA I/O In"=refnum<k21> "IO Socket\\SO 1 Serializer GPIO 2 Output") -> ()  [unwired: 1 out]
              n175 = xnode "FPGA I/O Node"("I/O Item"=w395, "FPGA I/O In"=refnum<k21> "IO Socket\\SO 1 Serializer GPIO 3 Output") -> ()  [unwired: 1 out]
            }
            frame "SO 2 Serializer" {
              n176 = xnode "FPGA I/O Node"("I/O Item"=w406, "FPGA I/O In"=refnum<k21> "IO Socket\\SO 2 Serializer GPIO 0 Output") -> ()  [unwired: 1 out]
              n177 = xnode "FPGA I/O Node"("I/O Item"=w405, "FPGA I/O In"=refnum<k21> "IO Socket\\SO 2 Serializer GPIO 1 Output") -> ()  [unwired: 1 out]
              n178 = xnode "FPGA I/O Node"("I/O Item"=w404, "FPGA I/O In"=refnum<k21> "IO Socket\\SO 2 Serializer GPIO 2 Output") -> ()  [unwired: 1 out]
              n179 = xnode "FPGA I/O Node"("I/O Item"=w403, "FPGA I/O In"=refnum<k21> "IO Socket\\SO 2 Serializer GPIO 3 Output") -> ()  [unwired: 1 out]
            }
            frame "SO 3 Serializer" {
              n180 = xnode "FPGA I/O Node"("I/O Item"=w414, "FPGA I/O In"=refnum<k21> "IO Socket\\SO 3 Serializer GPIO 0 Output") -> ()  [unwired: 1 out]
              n181 = xnode "FPGA I/O Node"("I/O Item"=w413, "FPGA I/O In"=refnum<k21> "IO Socket\\SO 3 Serializer GPIO 1 Output") -> ()  [unwired: 1 out]
              n182 = xnode "FPGA I/O Node"("I/O Item"=w412, "FPGA I/O In"=refnum<k21> "IO Socket\\SO 3 Serializer GPIO 2 Output") -> ()  [unwired: 1 out]
              n183 = xnode "FPGA I/O Node"("I/O Item"=w411, "FPGA I/O In"=refnum<k21> "IO Socket\\SO 3 Serializer GPIO 3 Output") -> ()  [unwired: 1 out]
            }
          }
          n184 = Not(x=w321) -> (.not. x?=w320:bool)
        }
        frame condition #5 {
          n185 = case shown="\"SI 3 Deserializer\"" w431 {
            tunnel: w430 -> [_ w445 w465 w485 w505 w516 w524 w532 w540]
            tunnel: w429 -> [_ w444 w464 w484 w504 w515 w523 w531 w539]
            tunnel: w428 -> [_ w443 w463 w483 w503 w514 w522 w530 w538]
            tunnel: w427 -> [_ w442 w462 w482 w502 w513 w521 w529 w537]
            tunnel: w426 -> [_ w441 w461 w481 w501 _ _ _ _]
            tunnel: w425 -> [_ w440 w460 w480 w500 _ _ _ _]
            tunnel: w424 -> [_ w439 w459 w479 w499 _ _ _ _]
            tunnel: [w432 _ _ _ _ _ _ _ _] -> w423
            tunnel: w421 -> [_ w435 w455 w473 w493 _ _ _ _]
            tunnel: w420 -> [_ w434 w454 w474 w494 _ _ _ _]
            tunnel: w419 -> [_ w433 w453 w475 w495 _ _ _ _]
            frame Default {
              w432 = TRUE  # serdes id invalid
            }
            frame "SI 0 Deserializer" {
              n186 = xnode "FPGA I/O Node"("I/O Item"=w445, "FPGA I/O In"=refnum<k21> "IO Socket\\SI 0 Deserializer GPIO 0 Output") -> ()  [unwired: 1 out]
              n187 = xnode "FPGA I/O Node"("I/O Item"=w444, "FPGA I/O In"=refnum<k21> "IO Socket\\SI 0 Deserializer GPIO 1 Output") -> ()  [unwired: 1 out]
              n188 = xnode "FPGA I/O Node"("I/O Item"=w443, "FPGA I/O In"=refnum<k21> "IO Socket\\SI 0 Deserializer GPIO 2 Output") -> ()  [unwired: 1 out]
              n189 = xnode "FPGA I/O Node"("I/O Item"=w442, "FPGA I/O In"=refnum<k21> "IO Socket\\SI 0 Deserializer GPIO 3 Output") -> ()  [unwired: 1 out]
              n190 = xnode "FPGA I/O Node"("I/O Item"=w441, "FPGA I/O In"=refnum<k21> "IO Socket\\SI 0 Deserializer GPIO 4 Output") -> ()  [unwired: 1 out]
              n191 = xnode "FPGA I/O Node"("I/O Item"=w440, "FPGA I/O In"=refnum<k21> "IO Socket\\SI 0 Deserializer GPIO 5 Output") -> ()  [unwired: 1 out]
              n192 = xnode "FPGA I/O Node"("I/O Item"=w439, "FPGA I/O In"=refnum<k21> "IO Socket\\SI 0 Deserializer GPIO 6 Output") -> ()  [unwired: 1 out]
              n193 = xnode "FPGA I/O Node"("I/O Item"=w435, "FPGA I/O In"=refnum<k21> "IO Socket\\SI 0 Deserializer GPIO 7 Output") -> ()  [unwired: 1 out]
              n194 = xnode "FPGA I/O Node"("I/O Item"=w434, "FPGA I/O In"=refnum<k21> "IO Socket\\SI 0 Deserializer GPIO 9 Output") -> ()  [unwired: 1 out]
              n195 = xnode "FPGA I/O Node"("I/O Item"=w433, "FPGA I/O In"=refnum<k21> "IO Socket\\SI 0 Deserializer GPIO 10 Output") -> ()  [unwired: 1 out]
            }
            frame "SI 1 Deserializer" {
              n196 = xnode "FPGA I/O Node"("I/O Item"=w465, "FPGA I/O In"=refnum<k21> "IO Socket\\SI 1 Deserializer GPIO 0 Output") -> ()  [unwired: 1 out]
              n197 = xnode "FPGA I/O Node"("I/O Item"=w464, "FPGA I/O In"=refnum<k21> "IO Socket\\SI 1 Deserializer GPIO 1 Output") -> ()  [unwired: 1 out]
              n198 = xnode "FPGA I/O Node"("I/O Item"=w463, "FPGA I/O In"=refnum<k21> "IO Socket\\SI 1 Deserializer GPIO 2 Output") -> ()  [unwired: 1 out]
              n199 = xnode "FPGA I/O Node"("I/O Item"=w462, "FPGA I/O In"=refnum<k21> "IO Socket\\SI 1 Deserializer GPIO 3 Output") -> ()  [unwired: 1 out]
              n200 = xnode "FPGA I/O Node"("I/O Item"=w461, "FPGA I/O In"=refnum<k21> "IO Socket\\SI 1 Deserializer GPIO 4 Output") -> ()  [unwired: 1 out]
              n201 = xnode "FPGA I/O Node"("I/O Item"=w460, "FPGA I/O In"=refnum<k21> "IO Socket\\SI 1 Deserializer GPIO 5 Output") -> ()  [unwired: 1 out]
              n202 = xnode "FPGA I/O Node"("I/O Item"=w459, "FPGA I/O In"=refnum<k21> "IO Socket\\SI 1 Deserializer GPIO 6 Output") -> ()  [unwired: 1 out]
              n203 = xnode "FPGA I/O Node"("I/O Item"=w455, "FPGA I/O In"=refnum<k21> "IO Socket\\SI 1 Deserializer GPIO 7 Output") -> ()  [unwired: 1 out]
              n204 = xnode "FPGA I/O Node"("I/O Item"=w454, "FPGA I/O In"=refnum<k21> "IO Socket\\SI 1 Deserializer GPIO 9 Output") -> ()  [unwired: 1 out]
              n205 = xnode "FPGA I/O Node"("I/O Item"=w453, "FPGA I/O In"=refnum<k21> "IO Socket\\SI 1 Deserializer GPIO 10 Output") -> ()  [unwired: 1 out]
            }
            frame "SI 2 Deserializer" {
              n206 = xnode "FPGA I/O Node"("I/O Item"=w485, "FPGA I/O In"=refnum<k21> "IO Socket\\SI 2 Deserializer GPIO 0 Output") -> ()  [unwired: 1 out]
              n207 = xnode "FPGA I/O Node"("I/O Item"=w484, "FPGA I/O In"=refnum<k21> "IO Socket\\SI 2 Deserializer GPIO 1 Output") -> ()  [unwired: 1 out]
              n208 = xnode "FPGA I/O Node"("I/O Item"=w483, "FPGA I/O In"=refnum<k21> "IO Socket\\SI 2 Deserializer GPIO 2 Output") -> ()  [unwired: 1 out]
              n209 = xnode "FPGA I/O Node"("I/O Item"=w482, "FPGA I/O In"=refnum<k21> "IO Socket\\SI 2 Deserializer GPIO 3 Output") -> ()  [unwired: 1 out]
              n210 = xnode "FPGA I/O Node"("I/O Item"=w481, "FPGA I/O In"=refnum<k21> "IO Socket\\SI 2 Deserializer GPIO 4 Output") -> ()  [unwired: 1 out]
              n211 = xnode "FPGA I/O Node"("I/O Item"=w480, "FPGA I/O In"=refnum<k21> "IO Socket\\SI 2 Deserializer GPIO 5 Output") -> ()  [unwired: 1 out]
              n212 = xnode "FPGA I/O Node"("I/O Item"=w479, "FPGA I/O In"=refnum<k21> "IO Socket\\SI 2 Deserializer GPIO 6 Output") -> ()  [unwired: 1 out]
              n213 = xnode "FPGA I/O Node"("I/O Item"=w473, "FPGA I/O In"=refnum<k21> "IO Socket\\SI 2 Deserializer GPIO 7 Output") -> ()  [unwired: 1 out]
              n214 = xnode "FPGA I/O Node"("I/O Item"=w474, "FPGA I/O In"=refnum<k21> "IO Socket\\SI 2 Deserializer GPIO 9 Output") -> ()  [unwired: 1 out]
              n215 = xnode "FPGA I/O Node"("I/O Item"=w475, "FPGA I/O In"=refnum<k21> "IO Socket\\SI 2 Deserializer GPIO 10 Output") -> ()  [unwired: 1 out]
            }
            frame "SI 3 Deserializer" {
              n216 = xnode "FPGA I/O Node"("I/O Item"=w505, "FPGA I/O In"=refnum<k21> "IO Socket\\SI 3 Deserializer GPIO 0 Output") -> ()  [unwired: 1 out]
              n217 = xnode "FPGA I/O Node"("I/O Item"=w504, "FPGA I/O In"=refnum<k21> "IO Socket\\SI 3 Deserializer GPIO 1 Output") -> ()  [unwired: 1 out]
              n218 = xnode "FPGA I/O Node"("I/O Item"=w503, "FPGA I/O In"=refnum<k21> "IO Socket\\SI 3 Deserializer GPIO 2 Output") -> ()  [unwired: 1 out]
              n219 = xnode "FPGA I/O Node"("I/O Item"=w502, "FPGA I/O In"=refnum<k21> "IO Socket\\SI 3 Deserializer GPIO 3 Output") -> ()  [unwired: 1 out]
              n220 = xnode "FPGA I/O Node"("I/O Item"=w501, "FPGA I/O In"=refnum<k21> "IO Socket\\SI 3 Deserializer GPIO 4 Output") -> ()  [unwired: 1 out]
              n221 = xnode "FPGA I/O Node"("I/O Item"=w500, "FPGA I/O In"=refnum<k21> "IO Socket\\SI 3 Deserializer GPIO 5 Output") -> ()  [unwired: 1 out]
              n222 = xnode "FPGA I/O Node"("I/O Item"=w499, "FPGA I/O In"=refnum<k21> "IO Socket\\SI 3 Deserializer GPIO 6 Output") -> ()  [unwired: 1 out]
              n223 = xnode "FPGA I/O Node"("I/O Item"=w493, "FPGA I/O In"=refnum<k21> "IO Socket\\SI 3 Deserializer GPIO 7 Output") -> ()  [unwired: 1 out]
              n224 = xnode "FPGA I/O Node"("I/O Item"=w494, "FPGA I/O In"=refnum<k21> "IO Socket\\SI 3 Deserializer GPIO 9 Output") -> ()  [unwired: 1 out]
              n225 = xnode "FPGA I/O Node"("I/O Item"=w495, "FPGA I/O In"=refnum<k21> "IO Socket\\SI 3 Deserializer GPIO 10 Output") -> ()  [unwired: 1 out]
            }
            frame "SO 0 Serializer" {
              n226 = xnode "FPGA I/O Node"("I/O Item"=w516, "FPGA I/O In"=refnum<k21> "IO Socket\\SO 0 Serializer GPIO 0 Output") -> ()  [unwired: 1 out]
              n227 = xnode "FPGA I/O Node"("I/O Item"=w515, "FPGA I/O In"=refnum<k21> "IO Socket\\SO 0 Serializer GPIO 1 Output") -> ()  [unwired: 1 out]
              n228 = xnode "FPGA I/O Node"("I/O Item"=w514, "FPGA I/O In"=refnum<k21> "IO Socket\\SO 0 Serializer GPIO 2 Output") -> ()  [unwired: 1 out]
              n229 = xnode "FPGA I/O Node"("I/O Item"=w513, "FPGA I/O In"=refnum<k21> "IO Socket\\SO 0 Serializer GPIO 3 Output") -> ()  [unwired: 1 out]
            }
            frame "SO 1 Serializer" {
              n230 = xnode "FPGA I/O Node"("I/O Item"=w524, "FPGA I/O In"=refnum<k21> "IO Socket\\SO 1 Serializer GPIO 0 Output") -> ()  [unwired: 1 out]
              n231 = xnode "FPGA I/O Node"("I/O Item"=w523, "FPGA I/O In"=refnum<k21> "IO Socket\\SO 1 Serializer GPIO 1 Output") -> ()  [unwired: 1 out]
              n232 = xnode "FPGA I/O Node"("I/O Item"=w522, "FPGA I/O In"=refnum<k21> "IO Socket\\SO 1 Serializer GPIO 2 Output") -> ()  [unwired: 1 out]
              n233 = xnode "FPGA I/O Node"("I/O Item"=w521, "FPGA I/O In"=refnum<k21> "IO Socket\\SO 1 Serializer GPIO 3 Output") -> ()  [unwired: 1 out]
            }
            frame "SO 2 Serializer" {
              n234 = xnode "FPGA I/O Node"("I/O Item"=w532, "FPGA I/O In"=refnum<k21> "IO Socket\\SO 2 Serializer GPIO 0 Output") -> ()  [unwired: 1 out]
              n235 = xnode "FPGA I/O Node"("I/O Item"=w531, "FPGA I/O In"=refnum<k21> "IO Socket\\SO 2 Serializer GPIO 1 Output") -> ()  [unwired: 1 out]
              n236 = xnode "FPGA I/O Node"("I/O Item"=w530, "FPGA I/O In"=refnum<k21> "IO Socket\\SO 2 Serializer GPIO 2 Output") -> ()  [unwired: 1 out]
              n237 = xnode "FPGA I/O Node"("I/O Item"=w529, "FPGA I/O In"=refnum<k21> "IO Socket\\SO 2 Serializer GPIO 3 Output") -> ()  [unwired: 1 out]
            }
            frame "SO 3 Serializer" {
              n238 = xnode "FPGA I/O Node"("I/O Item"=w540, "FPGA I/O In"=refnum<k21> "IO Socket\\SO 3 Serializer GPIO 0 Output") -> ()  [unwired: 1 out]
              n239 = xnode "FPGA I/O Node"("I/O Item"=w539, "FPGA I/O In"=refnum<k21> "IO Socket\\SO 3 Serializer GPIO 1 Output") -> ()  [unwired: 1 out]
              n240 = xnode "FPGA I/O Node"("I/O Item"=w538, "FPGA I/O In"=refnum<k21> "IO Socket\\SO 3 Serializer GPIO 2 Output") -> ()  [unwired: 1 out]
              n241 = xnode "FPGA I/O Node"("I/O Item"=w537, "FPGA I/O In"=refnum<k21> "IO Socket\\SO 3 Serializer GPIO 3 Output") -> ()  [unwired: 1 out]
            }
          }
          n242 = Not(x=w423) -> (.not. x?=w422:bool)
        }
        frame condition #6 {
          n243 = case shown="\"SI 0 SI 1 Deserializer\"" w558 {
            tunnel: w557 -> [_ w572 w590 w608 w626]
            tunnel: w556 -> [_ w571 w589 w607 w625]
            tunnel: w555 -> [_ _ _ _ _]
            tunnel: w554 -> [_ _ _ _ _]
            tunnel: w553 -> [_ w570 w588 w606 w624]
            tunnel: w552 -> [_ w569 w587 w605 w623]
            tunnel: w551 -> [_ w568 w586 w604 w622]
            tunnel: [w559 _ _ _ _] -> w550
            tunnel: w548 -> [_ w566 w584 w602 w620]
            tunnel: w547 -> [_ w562 w580 w598 w616]
            tunnel: w546 -> [_ w561 w579 w597 w615]
            tunnel: w545 -> [_ w560 w578 w596 w614]
            frame Default {
              w559 = TRUE  # serdes id invalid
            }
            frame "SI 0 SI 1 Deserializer" {
              n244 = xnode "FPGA I/O Node"("I/O Item"=w572, "FPGA I/O In"=refnum<k21> "IO Socket\\SI 0 SI 1 Deserializer MFP 0 Output") -> ()  [unwired: 1 out]
              n245 = xnode "FPGA I/O Node"("I/O Item"=w571, "FPGA I/O In"=refnum<k21> "IO Socket\\SI 0 SI 1 Deserializer MFP 1 Output") -> ()  [unwired: 1 out]
              n246 = xnode "FPGA I/O Node"("I/O Item"=w570, "FPGA I/O In"=refnum<k21> "IO Socket\\SI 0 SI 1 Deserializer MFP 4 Output") -> ()  [unwired: 1 out]
              n247 = xnode "FPGA I/O Node"("I/O Item"=w569, "FPGA I/O In"=refnum<k21> "IO Socket\\SI 0 SI 1 Deserializer MFP 5 Output") -> ()  [unwired: 1 out]
              n248 = xnode "FPGA I/O Node"("I/O Item"=w568, "FPGA I/O In"=refnum<k21> "IO Socket\\SI 0 SI 1 Deserializer MFP 6 Output") -> ()  [unwired: 1 out]
              n249 = xnode "FPGA I/O Node"("I/O Item"=w566, "FPGA I/O In"=refnum<k21> "IO Socket\\SI 0 SI 1 Deserializer MFP 7 Output") -> ()  [unwired: 1 out]
              n250 = xnode "FPGA I/O Node"("I/O Item"=w562, "FPGA I/O In"=refnum<k21> "IO Socket\\SI 0 SI 1 Deserializer MFP 8 Output") -> ()  [unwired: 1 out]
              n251 = xnode "FPGA I/O Node"("I/O Item"=w561, "FPGA I/O In"=refnum<k21> "IO Socket\\SI 0 SI 1 Deserializer MFP 9 Output") -> ()  [unwired: 1 out]
              n252 = xnode "FPGA I/O Node"("I/O Item"=w560, "FPGA I/O In"=refnum<k21> "IO Socket\\SI 0 SI 1 Deserializer MFP 10 Output") -> ()  [unwired: 1 out]
            }
            frame "SI 2 SI 3 Deserializer" {
              n253 = xnode "FPGA I/O Node"("I/O Item"=w590, "FPGA I/O In"=refnum<k21> "IO Socket\\SI 2 SI 3 Deserializer MFP 0 Output") -> ()  [unwired: 1 out]
              n254 = xnode "FPGA I/O Node"("I/O Item"=w589, "FPGA I/O In"=refnum<k21> "IO Socket\\SI 2 SI 3 Deserializer MFP 1 Output") -> ()  [unwired: 1 out]
              n255 = xnode "FPGA I/O Node"("I/O Item"=w588, "FPGA I/O In"=refnum<k21> "IO Socket\\SI 2 SI 3 Deserializer MFP 4 Output") -> ()  [unwired: 1 out]
              n256 = xnode "FPGA I/O Node"("I/O Item"=w587, "FPGA I/O In"=refnum<k21> "IO Socket\\SI 2 SI 3 Deserializer MFP 5 Output") -> ()  [unwired: 1 out]
              n257 = xnode "FPGA I/O Node"("I/O Item"=w586, "FPGA I/O In"=refnum<k21> "IO Socket\\SI 2 SI 3 Deserializer MFP 6 Output") -> ()  [unwired: 1 out]
              n258 = xnode "FPGA I/O Node"("I/O Item"=w584, "FPGA I/O In"=refnum<k21> "IO Socket\\SI 2 SI 3 Deserializer MFP 7 Output") -> ()  [unwired: 1 out]
              n259 = xnode "FPGA I/O Node"("I/O Item"=w580, "FPGA I/O In"=refnum<k21> "IO Socket\\SI 2 SI 3 Deserializer MFP 8 Output") -> ()  [unwired: 1 out]
              n260 = xnode "FPGA I/O Node"("I/O Item"=w579, "FPGA I/O In"=refnum<k21> "IO Socket\\SI 2 SI 3 Deserializer MFP 9 Output") -> ()  [unwired: 1 out]
              n261 = xnode "FPGA I/O Node"("I/O Item"=w578, "FPGA I/O In"=refnum<k21> "IO Socket\\SI 2 SI 3 Deserializer MFP 10 Output") -> ()  [unwired: 1 out]
            }
            frame "SI 4 SI 5 Deserializer" {
              n262 = xnode "FPGA I/O Node"("I/O Item"=w608, "FPGA I/O In"=refnum<k21> "IO Socket\\SI 4 SI 5 Deserializer MFP 0 Output") -> ()  [unwired: 1 out]
              n263 = xnode "FPGA I/O Node"("I/O Item"=w607, "FPGA I/O In"=refnum<k21> "IO Socket\\SI 4 SI 5 Deserializer MFP 1 Output") -> ()  [unwired: 1 out]
              n264 = xnode "FPGA I/O Node"("I/O Item"=w606, "FPGA I/O In"=refnum<k21> "IO Socket\\SI 4 SI 5 Deserializer MFP 4 Output") -> ()  [unwired: 1 out]
              n265 = xnode "FPGA I/O Node"("I/O Item"=w605, "FPGA I/O In"=refnum<k21> "IO Socket\\SI 4 SI 5 Deserializer MFP 5 Output") -> ()  [unwired: 1 out]
              n266 = xnode "FPGA I/O Node"("I/O Item"=w604, "FPGA I/O In"=refnum<k21> "IO Socket\\SI 4 SI 5 Deserializer MFP 6 Output") -> ()  [unwired: 1 out]
              n267 = xnode "FPGA I/O Node"("I/O Item"=w602, "FPGA I/O In"=refnum<k21> "IO Socket\\SI 4 SI 5 Deserializer MFP 7 Output") -> ()  [unwired: 1 out]
              n268 = xnode "FPGA I/O Node"("I/O Item"=w598, "FPGA I/O In"=refnum<k21> "IO Socket\\SI 4 SI 5 Deserializer MFP 8 Output") -> ()  [unwired: 1 out]
              n269 = xnode "FPGA I/O Node"("I/O Item"=w597, "FPGA I/O In"=refnum<k21> "IO Socket\\SI 4 SI 5 Deserializer MFP 9 Output") -> ()  [unwired: 1 out]
              n270 = xnode "FPGA I/O Node"("I/O Item"=w596, "FPGA I/O In"=refnum<k21> "IO Socket\\SI 4 SI 5 Deserializer MFP 10 Output") -> ()  [unwired: 1 out]
            }
            frame "SI 6 SI 7 Deserializer" {
              n271 = xnode "FPGA I/O Node"("I/O Item"=w626, "FPGA I/O In"=refnum<k21> "IO Socket\\SI 6 SI 7 Deserializer MFP 0 Output") -> ()  [unwired: 1 out]
              n272 = xnode "FPGA I/O Node"("I/O Item"=w625, "FPGA I/O In"=refnum<k21> "IO Socket\\SI 6 SI 7 Deserializer MFP 1 Output") -> ()  [unwired: 1 out]
              n273 = xnode "FPGA I/O Node"("I/O Item"=w624, "FPGA I/O In"=refnum<k21> "IO Socket\\SI 6 SI 7 Deserializer MFP 4 Output") -> ()  [unwired: 1 out]
              n274 = xnode "FPGA I/O Node"("I/O Item"=w623, "FPGA I/O In"=refnum<k21> "IO Socket\\SI 6 SI 7 Deserializer MFP 5 Output") -> ()  [unwired: 1 out]
              n275 = xnode "FPGA I/O Node"("I/O Item"=w622, "FPGA I/O In"=refnum<k21> "IO Socket\\SI 6 SI 7 Deserializer MFP 6 Output") -> ()  [unwired: 1 out]
              n276 = xnode "FPGA I/O Node"("I/O Item"=w620, "FPGA I/O In"=refnum<k21> "IO Socket\\SI 6 SI 7 Deserializer MFP 7 Output") -> ()  [unwired: 1 out]
              n277 = xnode "FPGA I/O Node"("I/O Item"=w616, "FPGA I/O In"=refnum<k21> "IO Socket\\SI 6 SI 7 Deserializer MFP 8 Output") -> ()  [unwired: 1 out]
              n278 = xnode "FPGA I/O Node"("I/O Item"=w615, "FPGA I/O In"=refnum<k21> "IO Socket\\SI 6 SI 7 Deserializer MFP 9 Output") -> ()  [unwired: 1 out]
              n279 = xnode "FPGA I/O Node"("I/O Item"=w614, "FPGA I/O In"=refnum<k21> "IO Socket\\SI 6 SI 7 Deserializer MFP 10 Output") -> ()  [unwired: 1 out]
            }
          }
          n280 = Not(x=w550) -> (.not. x?=w549:bool)
        }
        frame condition #7 {
          n281 = case shown="\"SI 0 SI 1 Deserializer\"" w645 {
            tunnel: w644 -> [_ w659 w677]
            tunnel: w643 -> [_ w658 w676]
            tunnel: w642 -> [_ _ _]
            tunnel: w641 -> [_ _ _]
            tunnel: w640 -> [_ w657 w675]
            tunnel: w639 -> [_ w656 w674]
            tunnel: w638 -> [_ w655 w673]
            tunnel: [w646 _ _] -> w637
            tunnel: w635 -> [_ w653 w671]
            tunnel: w634 -> [_ w649 w667]
            tunnel: w633 -> [_ w648 w666]
            tunnel: w632 -> [_ w647 w665]
            frame Default {
              w646 = TRUE  # serdes id invalid
            }
            frame "SI 0 SI 1 Deserializer" {
              n282 = xnode "FPGA I/O Node"("I/O Item"=w659, "FPGA I/O In"=refnum<k21> "IO Socket\\SI 0 SI 1 Deserializer MFP 0 Output") -> ()  [unwired: 1 out]
              n283 = xnode "FPGA I/O Node"("I/O Item"=w658, "FPGA I/O In"=refnum<k21> "IO Socket\\SI 0 SI 1 Deserializer MFP 1 Output") -> ()  [unwired: 1 out]
              n284 = xnode "FPGA I/O Node"("I/O Item"=w657, "FPGA I/O In"=refnum<k21> "IO Socket\\SI 0 SI 1 Deserializer MFP 4 Output") -> ()  [unwired: 1 out]
              n285 = xnode "FPGA I/O Node"("I/O Item"=w656, "FPGA I/O In"=refnum<k21> "IO Socket\\SI 0 SI 1 Deserializer MFP 5 Output") -> ()  [unwired: 1 out]
              n286 = xnode "FPGA I/O Node"("I/O Item"=w655, "FPGA I/O In"=refnum<k21> "IO Socket\\SI 0 SI 1 Deserializer MFP 6 Output") -> ()  [unwired: 1 out]
              n287 = xnode "FPGA I/O Node"("I/O Item"=w653, "FPGA I/O In"=refnum<k21> "IO Socket\\SI 0 SI 1 Deserializer MFP 7 Output") -> ()  [unwired: 1 out]
              n288 = xnode "FPGA I/O Node"("I/O Item"=w649, "FPGA I/O In"=refnum<k21> "IO Socket\\SI 0 SI 1 Deserializer MFP 8 Output") -> ()  [unwired: 1 out]
              n289 = xnode "FPGA I/O Node"("I/O Item"=w648, "FPGA I/O In"=refnum<k21> "IO Socket\\SI 0 SI 1 Deserializer MFP 9 Output") -> ()  [unwired: 1 out]
              n290 = xnode "FPGA I/O Node"("I/O Item"=w647, "FPGA I/O In"=refnum<k21> "IO Socket\\SI 0 SI 1 Deserializer MFP 10 Output") -> ()  [unwired: 1 out]
            }
            frame "SI 2 SI 3 Deserializer" {
              n291 = xnode "FPGA I/O Node"("I/O Item"=w677, "FPGA I/O In"=refnum<k21> "IO Socket\\SI 2 SI 3 Deserializer MFP 0 Output") -> ()  [unwired: 1 out]
              n292 = xnode "FPGA I/O Node"("I/O Item"=w676, "FPGA I/O In"=refnum<k21> "IO Socket\\SI 2 SI 3 Deserializer MFP 1 Output") -> ()  [unwired: 1 out]
              n293 = xnode "FPGA I/O Node"("I/O Item"=w675, "FPGA I/O In"=refnum<k21> "IO Socket\\SI 2 SI 3 Deserializer MFP 4 Output") -> ()  [unwired: 1 out]
              n294 = xnode "FPGA I/O Node"("I/O Item"=w674, "FPGA I/O In"=refnum<k21> "IO Socket\\SI 2 SI 3 Deserializer MFP 5 Output") -> ()  [unwired: 1 out]
              n295 = xnode "FPGA I/O Node"("I/O Item"=w673, "FPGA I/O In"=refnum<k21> "IO Socket\\SI 2 SI 3 Deserializer MFP 6 Output") -> ()  [unwired: 1 out]
              n296 = xnode "FPGA I/O Node"("I/O Item"=w671, "FPGA I/O In"=refnum<k21> "IO Socket\\SI 2 SI 3 Deserializer MFP 7 Output") -> ()  [unwired: 1 out]
              n297 = xnode "FPGA I/O Node"("I/O Item"=w667, "FPGA I/O In"=refnum<k21> "IO Socket\\SI 2 SI 3 Deserializer MFP 8 Output") -> ()  [unwired: 1 out]
              n298 = xnode "FPGA I/O Node"("I/O Item"=w666, "FPGA I/O In"=refnum<k21> "IO Socket\\SI 2 SI 3 Deserializer MFP 9 Output") -> ()  [unwired: 1 out]
              n299 = xnode "FPGA I/O Node"("I/O Item"=w665, "FPGA I/O In"=refnum<k21> "IO Socket\\SI 2 SI 3 Deserializer MFP 10 Output") -> ()  [unwired: 1 out]
            }
          }
          n300 = Not(x=w637) -> (.not. x?=w636:bool)
        }
        frame condition #8 {
          n301 = case shown="\"SO 7 Serializer\"" w691 {
            tunnel: w690 -> [_ w702 w714 w726 w738 w750 w762 w774 w786]
            tunnel: w689 -> [_ w701 w713 w725 w737 w749 w761 w773 w785]
            tunnel: w688 -> [_ w697 w709 w721 w733 w745 w757 w769 w781]
            tunnel: w687 -> [_ w696 w708 w720 w732 w744 w756 w768 w780]
            tunnel: [w692 _ _ _ _ _ _ _ _] -> w686
            tunnel: w684 -> [_ w695 w707 w719 w731 w743 w755 w767 w779]
            tunnel: w683 -> [_ w693 w705 w717 w729 w741 w753 w765 w777]
            frame Default {
              w692 = TRUE  # serdes id invalid
            }
            frame "SO 0 Serializer" {
              n302 = xnode "FPGA I/O Node"("I/O Item"=w702, "FPGA I/O In"=refnum<k21> "IO Socket\\SO 0 Serializer MFP 0 Output") -> ()  [unwired: 1 out]
              n303 = xnode "FPGA I/O Node"("I/O Item"=w701, "FPGA I/O In"=refnum<k21> "IO Socket\\SO 0 Serializer MFP 3 Output") -> ()  [unwired: 1 out]
              n304 = xnode "FPGA I/O Node"("I/O Item"=w697, "FPGA I/O In"=refnum<k21> "IO Socket\\SO 0 Serializer MFP 4 Output") -> ()  [unwired: 1 out]
              n305 = xnode "FPGA I/O Node"("I/O Item"=w696, "FPGA I/O In"=refnum<k21> "IO Socket\\SO 0 Serializer MFP 6 Output") -> ()  [unwired: 1 out]
              n306 = xnode "FPGA I/O Node"("I/O Item"=w695, "FPGA I/O In"=refnum<k21> "IO Socket\\SO 0 Serializer MFP 7 Output") -> ()  [unwired: 1 out]
              n307 = xnode "FPGA I/O Node"("I/O Item"=w693, "FPGA I/O In"=refnum<k21> "IO Socket\\SO 0 Serializer MFP 8 Output") -> ()  [unwired: 1 out]
            }
            frame "SO 1 Serializer" {
              n308 = xnode "FPGA I/O Node"("I/O Item"=w714, "FPGA I/O In"=refnum<k21> "IO Socket\\SO 1 Serializer MFP 0 Output") -> ()  [unwired: 1 out]
              n309 = xnode "FPGA I/O Node"("I/O Item"=w713, "FPGA I/O In"=refnum<k21> "IO Socket\\SO 1 Serializer MFP 3 Output") -> ()  [unwired: 1 out]
              n310 = xnode "FPGA I/O Node"("I/O Item"=w709, "FPGA I/O In"=refnum<k21> "IO Socket\\SO 1 Serializer MFP 4 Output") -> ()  [unwired: 1 out]
              n311 = xnode "FPGA I/O Node"("I/O Item"=w708, "FPGA I/O In"=refnum<k21> "IO Socket\\SO 1 Serializer MFP 6 Output") -> ()  [unwired: 1 out]
              n312 = xnode "FPGA I/O Node"("I/O Item"=w707, "FPGA I/O In"=refnum<k21> "IO Socket\\SO 1 Serializer MFP 7 Output") -> ()  [unwired: 1 out]
              n313 = xnode "FPGA I/O Node"("I/O Item"=w705, "FPGA I/O In"=refnum<k21> "IO Socket\\SO 1 Serializer MFP 8 Output") -> ()  [unwired: 1 out]
            }
            frame "SO 2 Serializer" {
              n314 = xnode "FPGA I/O Node"("I/O Item"=w726, "FPGA I/O In"=refnum<k21> "IO Socket\\SO 2 Serializer MFP 0 Output") -> ()  [unwired: 1 out]
              n315 = xnode "FPGA I/O Node"("I/O Item"=w725, "FPGA I/O In"=refnum<k21> "IO Socket\\SO 2 Serializer MFP 3 Output") -> ()  [unwired: 1 out]
              n316 = xnode "FPGA I/O Node"("I/O Item"=w721, "FPGA I/O In"=refnum<k21> "IO Socket\\SO 2 Serializer MFP 4 Output") -> ()  [unwired: 1 out]
              n317 = xnode "FPGA I/O Node"("I/O Item"=w720, "FPGA I/O In"=refnum<k21> "IO Socket\\SO 2 Serializer MFP 6 Output") -> ()  [unwired: 1 out]
              n318 = xnode "FPGA I/O Node"("I/O Item"=w719, "FPGA I/O In"=refnum<k21> "IO Socket\\SO 2 Serializer MFP 7 Output") -> ()  [unwired: 1 out]
              n319 = xnode "FPGA I/O Node"("I/O Item"=w717, "FPGA I/O In"=refnum<k21> "IO Socket\\SO 2 Serializer MFP 8 Output") -> ()  [unwired: 1 out]
            }
            frame "SO 3 Serializer" {
              n320 = xnode "FPGA I/O Node"("I/O Item"=w738, "FPGA I/O In"=refnum<k21> "IO Socket\\SO 3 Serializer MFP 0 Output") -> ()  [unwired: 1 out]
              n321 = xnode "FPGA I/O Node"("I/O Item"=w737, "FPGA I/O In"=refnum<k21> "IO Socket\\SO 3 Serializer MFP 3 Output") -> ()  [unwired: 1 out]
              n322 = xnode "FPGA I/O Node"("I/O Item"=w733, "FPGA I/O In"=refnum<k21> "IO Socket\\SO 3 Serializer MFP 4 Output") -> ()  [unwired: 1 out]
              n323 = xnode "FPGA I/O Node"("I/O Item"=w732, "FPGA I/O In"=refnum<k21> "IO Socket\\SO 3 Serializer MFP 6 Output") -> ()  [unwired: 1 out]
              n324 = xnode "FPGA I/O Node"("I/O Item"=w731, "FPGA I/O In"=refnum<k21> "IO Socket\\SO 3 Serializer MFP 7 Output") -> ()  [unwired: 1 out]
              n325 = xnode "FPGA I/O Node"("I/O Item"=w729, "FPGA I/O In"=refnum<k21> "IO Socket\\SO 3 Serializer MFP 8 Output") -> ()  [unwired: 1 out]
            }
            frame "SO 4 Serializer" {
              n326 = xnode "FPGA I/O Node"("I/O Item"=w750, "FPGA I/O In"=refnum<k21> "IO Socket\\SO 4 Serializer MFP 0 Output") -> ()  [unwired: 1 out]
              n327 = xnode "FPGA I/O Node"("I/O Item"=w749, "FPGA I/O In"=refnum<k21> "IO Socket\\SO 4 Serializer MFP 3 Output") -> ()  [unwired: 1 out]
              n328 = xnode "FPGA I/O Node"("I/O Item"=w745, "FPGA I/O In"=refnum<k21> "IO Socket\\SO 4 Serializer MFP 4 Output") -> ()  [unwired: 1 out]
              n329 = xnode "FPGA I/O Node"("I/O Item"=w744, "FPGA I/O In"=refnum<k21> "IO Socket\\SO 4 Serializer MFP 6 Output") -> ()  [unwired: 1 out]
              n330 = xnode "FPGA I/O Node"("I/O Item"=w743, "FPGA I/O In"=refnum<k21> "IO Socket\\SO 4 Serializer MFP 7 Output") -> ()  [unwired: 1 out]
              n331 = xnode "FPGA I/O Node"("I/O Item"=w741, "FPGA I/O In"=refnum<k21> "IO Socket\\SO 4 Serializer MFP 8 Output") -> ()  [unwired: 1 out]
            }
            frame "SO 5 Serializer" {
              n332 = xnode "FPGA I/O Node"("I/O Item"=w762, "FPGA I/O In"=refnum<k21> "IO Socket\\SO 5 Serializer MFP 0 Output") -> ()  [unwired: 1 out]
              n333 = xnode "FPGA I/O Node"("I/O Item"=w761, "FPGA I/O In"=refnum<k21> "IO Socket\\SO 5 Serializer MFP 3 Output") -> ()  [unwired: 1 out]
              n334 = xnode "FPGA I/O Node"("I/O Item"=w757, "FPGA I/O In"=refnum<k21> "IO Socket\\SO 5 Serializer MFP 4 Output") -> ()  [unwired: 1 out]
              n335 = xnode "FPGA I/O Node"("I/O Item"=w756, "FPGA I/O In"=refnum<k21> "IO Socket\\SO 5 Serializer MFP 6 Output") -> ()  [unwired: 1 out]
              n336 = xnode "FPGA I/O Node"("I/O Item"=w755, "FPGA I/O In"=refnum<k21> "IO Socket\\SO 5 Serializer MFP 7 Output") -> ()  [unwired: 1 out]
              n337 = xnode "FPGA I/O Node"("I/O Item"=w753, "FPGA I/O In"=refnum<k21> "IO Socket\\SO 5 Serializer MFP 8 Output") -> ()  [unwired: 1 out]
            }
            frame "SO 6 Serializer" {
              n338 = xnode "FPGA I/O Node"("I/O Item"=w774, "FPGA I/O In"=refnum<k21> "IO Socket\\SO 6 Serializer MFP 0 Output") -> ()  [unwired: 1 out]
              n339 = xnode "FPGA I/O Node"("I/O Item"=w773, "FPGA I/O In"=refnum<k21> "IO Socket\\SO 6 Serializer MFP 3 Output") -> ()  [unwired: 1 out]
              n340 = xnode "FPGA I/O Node"("I/O Item"=w769, "FPGA I/O In"=refnum<k21> "IO Socket\\SO 6 Serializer MFP 4 Output") -> ()  [unwired: 1 out]
              n341 = xnode "FPGA I/O Node"("I/O Item"=w768, "FPGA I/O In"=refnum<k21> "IO Socket\\SO 6 Serializer MFP 6 Output") -> ()  [unwired: 1 out]
              n342 = xnode "FPGA I/O Node"("I/O Item"=w767, "FPGA I/O In"=refnum<k21> "IO Socket\\SO 6 Serializer MFP 7 Output") -> ()  [unwired: 1 out]
              n343 = xnode "FPGA I/O Node"("I/O Item"=w765, "FPGA I/O In"=refnum<k21> "IO Socket\\SO 6 Serializer MFP 8 Output") -> ()  [unwired: 1 out]
            }
            frame "SO 7 Serializer" {
              n344 = xnode "FPGA I/O Node"("I/O Item"=w786, "FPGA I/O In"=refnum<k21> "IO Socket\\SO 7 Serializer MFP 0 Output") -> ()  [unwired: 1 out]
              n345 = xnode "FPGA I/O Node"("I/O Item"=w785, "FPGA I/O In"=refnum<k21> "IO Socket\\SO 7 Serializer MFP 3 Output") -> ()  [unwired: 1 out]
              n346 = xnode "FPGA I/O Node"("I/O Item"=w781, "FPGA I/O In"=refnum<k21> "IO Socket\\SO 7 Serializer MFP 4 Output") -> ()  [unwired: 1 out]
              n347 = xnode "FPGA I/O Node"("I/O Item"=w780, "FPGA I/O In"=refnum<k21> "IO Socket\\SO 7 Serializer MFP 6 Output") -> ()  [unwired: 1 out]
              n348 = xnode "FPGA I/O Node"("I/O Item"=w779, "FPGA I/O In"=refnum<k21> "IO Socket\\SO 7 Serializer MFP 7 Output") -> ()  [unwired: 1 out]
              n349 = xnode "FPGA I/O Node"("I/O Item"=w777, "FPGA I/O In"=refnum<k21> "IO Socket\\SO 7 Serializer MFP 8 Output") -> ()  [unwired: 1 out]
            }
          }
          n350 = Not(x=w686) -> (.not. x?=w685:bool)
        }
        frame condition #9 {
          n351 = case shown="\"SO 3 Serializer\"" w797 {
            tunnel: w796 -> [_ w808 w820 w832 w844]
            tunnel: w795 -> [_ w807 w819 w831 w843]
            tunnel: w794 -> [_ w803 w815 w827 w839]
            tunnel: w793 -> [_ w802 w814 w826 w838]
            tunnel: [w798 _ _ _ _] -> w792
            tunnel: w790 -> [_ w801 w813 w825 w837]
            tunnel: w789 -> [_ w799 w811 w823 w835]
            frame Default {
              w798 = TRUE  # serdes id invalid
            }
            frame "SO 0 Serializer" {
              n352 = xnode "FPGA I/O Node"("I/O Item"=w808, "FPGA I/O In"=refnum<k21> "IO Socket\\SO 0 Serializer MFP 0 Output") -> ()  [unwired: 1 out]
              n353 = xnode "FPGA I/O Node"("I/O Item"=w807, "FPGA I/O In"=refnum<k21> "IO Socket\\SO 0 Serializer MFP 3 Output") -> ()  [unwired: 1 out]
              n354 = xnode "FPGA I/O Node"("I/O Item"=w803, "FPGA I/O In"=refnum<k21> "IO Socket\\SO 0 Serializer MFP 4 Output") -> ()  [unwired: 1 out]
              n355 = xnode "FPGA I/O Node"("I/O Item"=w802, "FPGA I/O In"=refnum<k21> "IO Socket\\SO 0 Serializer MFP 6 Output") -> ()  [unwired: 1 out]
              n356 = xnode "FPGA I/O Node"("I/O Item"=w801, "FPGA I/O In"=refnum<k21> "IO Socket\\SO 0 Serializer MFP 7 Output") -> ()  [unwired: 1 out]
              n357 = xnode "FPGA I/O Node"("I/O Item"=w799, "FPGA I/O In"=refnum<k21> "IO Socket\\SO 0 Serializer MFP 8 Output") -> ()  [unwired: 1 out]
            }
            frame "SO 1 Serializer" {
              n358 = xnode "FPGA I/O Node"("I/O Item"=w820, "FPGA I/O In"=refnum<k21> "IO Socket\\SO 1 Serializer MFP 0 Output") -> ()  [unwired: 1 out]
              n359 = xnode "FPGA I/O Node"("I/O Item"=w819, "FPGA I/O In"=refnum<k21> "IO Socket\\SO 1 Serializer MFP 3 Output") -> ()  [unwired: 1 out]
              n360 = xnode "FPGA I/O Node"("I/O Item"=w815, "FPGA I/O In"=refnum<k21> "IO Socket\\SO 1 Serializer MFP 4 Output") -> ()  [unwired: 1 out]
              n361 = xnode "FPGA I/O Node"("I/O Item"=w814, "FPGA I/O In"=refnum<k21> "IO Socket\\SO 1 Serializer MFP 6 Output") -> ()  [unwired: 1 out]
              n362 = xnode "FPGA I/O Node"("I/O Item"=w813, "FPGA I/O In"=refnum<k21> "IO Socket\\SO 1 Serializer MFP 7 Output") -> ()  [unwired: 1 out]
              n363 = xnode "FPGA I/O Node"("I/O Item"=w811, "FPGA I/O In"=refnum<k21> "IO Socket\\SO 1 Serializer MFP 8 Output") -> ()  [unwired: 1 out]
            }
            frame "SO 2 Serializer" {
              n364 = xnode "FPGA I/O Node"("I/O Item"=w832, "FPGA I/O In"=refnum<k21> "IO Socket\\SO 2 Serializer MFP 0 Output") -> ()  [unwired: 1 out]
              n365 = xnode "FPGA I/O Node"("I/O Item"=w831, "FPGA I/O In"=refnum<k21> "IO Socket\\SO 2 Serializer MFP 3 Output") -> ()  [unwired: 1 out]
              n366 = xnode "FPGA I/O Node"("I/O Item"=w827, "FPGA I/O In"=refnum<k21> "IO Socket\\SO 2 Serializer MFP 4 Output") -> ()  [unwired: 1 out]
              n367 = xnode "FPGA I/O Node"("I/O Item"=w826, "FPGA I/O In"=refnum<k21> "IO Socket\\SO 2 Serializer MFP 6 Output") -> ()  [unwired: 1 out]
              n368 = xnode "FPGA I/O Node"("I/O Item"=w825, "FPGA I/O In"=refnum<k21> "IO Socket\\SO 2 Serializer MFP 7 Output") -> ()  [unwired: 1 out]
              n369 = xnode "FPGA I/O Node"("I/O Item"=w823, "FPGA I/O In"=refnum<k21> "IO Socket\\SO 2 Serializer MFP 8 Output") -> ()  [unwired: 1 out]
            }
            frame "SO 3 Serializer" {
              n370 = xnode "FPGA I/O Node"("I/O Item"=w844, "FPGA I/O In"=refnum<k21> "IO Socket\\SO 3 Serializer MFP 0 Output") -> ()  [unwired: 1 out]
              n371 = xnode "FPGA I/O Node"("I/O Item"=w843, "FPGA I/O In"=refnum<k21> "IO Socket\\SO 3 Serializer MFP 3 Output") -> ()  [unwired: 1 out]
              n372 = xnode "FPGA I/O Node"("I/O Item"=w839, "FPGA I/O In"=refnum<k21> "IO Socket\\SO 3 Serializer MFP 4 Output") -> ()  [unwired: 1 out]
              n373 = xnode "FPGA I/O Node"("I/O Item"=w838, "FPGA I/O In"=refnum<k21> "IO Socket\\SO 3 Serializer MFP 6 Output") -> ()  [unwired: 1 out]
              n374 = xnode "FPGA I/O Node"("I/O Item"=w837, "FPGA I/O In"=refnum<k21> "IO Socket\\SO 3 Serializer MFP 7 Output") -> ()  [unwired: 1 out]
              n375 = xnode "FPGA I/O Node"("I/O Item"=w835, "FPGA I/O In"=refnum<k21> "IO Socket\\SO 3 Serializer MFP 8 Output") -> ()  [unwired: 1 out]
            }
          }
          n376 = Not(x=w792) -> (.not. x?=w791:bool)
        }
        frame condition #10 {
          n377 = case shown="\"SI 2 Deserializer\"" w860 {
            tunnel: w859 -> [_ w874 w892 w910 w928 w943 w955 w967 w979]
            tunnel: w858 -> [_ w873 w891 w909 w927 _ _ _ _]
            tunnel: w857 -> [_ _ _ _ _ _ _ _ _]
            tunnel: w856 -> [_ _ _ _ _ w942 w954 w966 w978]
            tunnel: w855 -> [_ w872 w890 w908 w926 w938 w950 w962 w974]
            tunnel: w854 -> [_ w871 w889 w907 w925 _ _ _ _]
            tunnel: w853 -> [_ w870 w888 w906 w924 w937 w949 w961 w973]
            tunnel: [w861 _ _ _ _ _ _ _ _] -> w852
            tunnel: w850 -> [_ w862 w880 w898 w916 w936 w948 w960 w972]
            tunnel: w849 -> [_ w863 w881 w899 w917 w934 w946 w958 w970]
            tunnel: w848 -> [_ w864 w882 w900 w918 _ _ _ _]
            tunnel: w847 -> [_ w865 w883 w901 w919 _ _ _ _]
            frame Default {
              w861 = TRUE  # serdes id invalid
            }
            frame "SI 0 Deserializer" {
              n378 = xnode "FPGA I/O Node"("I/O Item"=w874, "FPGA I/O In"=refnum<k21> "IO Socket\\SI 0 Deserializer MFP 0 Output") -> ()  [unwired: 1 out]
              n379 = xnode "FPGA I/O Node"("I/O Item"=w873, "FPGA I/O In"=refnum<k21> "IO Socket\\SI 0 Deserializer MFP 1 Output") -> ()  [unwired: 1 out]
              n380 = xnode "FPGA I/O Node"("I/O Item"=w872, "FPGA I/O In"=refnum<k21> "IO Socket\\SI 0 Deserializer MFP 4 Output") -> ()  [unwired: 1 out]
              n381 = xnode "FPGA I/O Node"("I/O Item"=w871, "FPGA I/O In"=refnum<k21> "IO Socket\\SI 0 Deserializer MFP 5 Output") -> ()  [unwired: 1 out]
              n382 = xnode "FPGA I/O Node"("I/O Item"=w870, "FPGA I/O In"=refnum<k21> "IO Socket\\SI 0 Deserializer MFP 6 Output") -> ()  [unwired: 1 out]
              n383 = xnode "FPGA I/O Node"("I/O Item"=w862, "FPGA I/O In"=refnum<k21> "IO Socket\\SI 0 Deserializer MFP 7 Output") -> ()  [unwired: 1 out]
              n384 = xnode "FPGA I/O Node"("I/O Item"=w863, "FPGA I/O In"=refnum<k21> "IO Socket\\SI 0 Deserializer MFP 8 Output") -> ()  [unwired: 1 out]
              n385 = xnode "FPGA I/O Node"("I/O Item"=w864, "FPGA I/O In"=refnum<k21> "IO Socket\\SI 0 Deserializer MFP 9 Output") -> ()  [unwired: 1 out]
              n386 = xnode "FPGA I/O Node"("I/O Item"=w865, "FPGA I/O In"=refnum<k21> "IO Socket\\SI 0 Deserializer MFP 10 Output") -> ()  [unwired: 1 out]
            }
            frame "SI 1 Deserializer" {
              n387 = xnode "FPGA I/O Node"("I/O Item"=w892, "FPGA I/O In"=refnum<k21> "IO Socket\\SI 1 Deserializer MFP 0 Output") -> ()  [unwired: 1 out]
              n388 = xnode "FPGA I/O Node"("I/O Item"=w891, "FPGA I/O In"=refnum<k21> "IO Socket\\SI 1 Deserializer MFP 1 Output") -> ()  [unwired: 1 out]
              n389 = xnode "FPGA I/O Node"("I/O Item"=w890, "FPGA I/O In"=refnum<k21> "IO Socket\\SI 1 Deserializer MFP 4 Output") -> ()  [unwired: 1 out]
              n390 = xnode "FPGA I/O Node"("I/O Item"=w889, "FPGA I/O In"=refnum<k21> "IO Socket\\SI 1 Deserializer MFP 5 Output") -> ()  [unwired: 1 out]
              n391 = xnode "FPGA I/O Node"("I/O Item"=w888, "FPGA I/O In"=refnum<k21> "IO Socket\\SI 1 Deserializer MFP 6 Output") -> ()  [unwired: 1 out]
              n392 = xnode "FPGA I/O Node"("I/O Item"=w880, "FPGA I/O In"=refnum<k21> "IO Socket\\SI 1 Deserializer MFP 7 Output") -> ()  [unwired: 1 out]
              n393 = xnode "FPGA I/O Node"("I/O Item"=w881, "FPGA I/O In"=refnum<k21> "IO Socket\\SI 1 Deserializer MFP 8 Output") -> ()  [unwired: 1 out]
              n394 = xnode "FPGA I/O Node"("I/O Item"=w882, "FPGA I/O In"=refnum<k21> "IO Socket\\SI 1 Deserializer MFP 9 Output") -> ()  [unwired: 1 out]
              n395 = xnode "FPGA I/O Node"("I/O Item"=w883, "FPGA I/O In"=refnum<k21> "IO Socket\\SI 1 Deserializer MFP 10 Output") -> ()  [unwired: 1 out]
            }
            frame "SI 2 Deserializer" {
              n396 = xnode "FPGA I/O Node"("I/O Item"=w910, "FPGA I/O In"=refnum<k21> "IO Socket\\SI 2 Deserializer MFP 0 Output") -> ()  [unwired: 1 out]
              n397 = xnode "FPGA I/O Node"("I/O Item"=w909, "FPGA I/O In"=refnum<k21> "IO Socket\\SI 2 Deserializer MFP 1 Output") -> ()  [unwired: 1 out]
              n398 = xnode "FPGA I/O Node"("I/O Item"=w908, "FPGA I/O In"=refnum<k21> "IO Socket\\SI 2 Deserializer MFP 4 Output") -> ()  [unwired: 1 out]
              n399 = xnode "FPGA I/O Node"("I/O Item"=w907, "FPGA I/O In"=refnum<k21> "IO Socket\\SI 2 Deserializer MFP 5 Output") -> ()  [unwired: 1 out]
              n400 = xnode "FPGA I/O Node"("I/O Item"=w906, "FPGA I/O In"=refnum<k21> "IO Socket\\SI 2 Deserializer MFP 6 Output") -> ()  [unwired: 1 out]
              n401 = xnode "FPGA I/O Node"("I/O Item"=w898, "FPGA I/O In"=refnum<k21> "IO Socket\\SI 2 Deserializer MFP 7 Output") -> ()  [unwired: 1 out]
              n402 = xnode "FPGA I/O Node"("I/O Item"=w899, "FPGA I/O In"=refnum<k21> "IO Socket\\SI 2 Deserializer MFP 8 Output") -> ()  [unwired: 1 out]
              n403 = xnode "FPGA I/O Node"("I/O Item"=w900, "FPGA I/O In"=refnum<k21> "IO Socket\\SI 2 Deserializer MFP 9 Output") -> ()  [unwired: 1 out]
              n404 = xnode "FPGA I/O Node"("I/O Item"=w901, "FPGA I/O In"=refnum<k21> "IO Socket\\SI 2 Deserializer MFP 10 Output") -> ()  [unwired: 1 out]
            }
            frame "SI 3 Deserializer" {
              n405 = xnode "FPGA I/O Node"("I/O Item"=w928, "FPGA I/O In"=refnum<k21> "IO Socket\\SI 3 Deserializer MFP 0 Output") -> ()  [unwired: 1 out]
              n406 = xnode "FPGA I/O Node"("I/O Item"=w927, "FPGA I/O In"=refnum<k21> "IO Socket\\SI 3 Deserializer MFP 1 Output") -> ()  [unwired: 1 out]
              n407 = xnode "FPGA I/O Node"("I/O Item"=w926, "FPGA I/O In"=refnum<k21> "IO Socket\\SI 3 Deserializer MFP 4 Output") -> ()  [unwired: 1 out]
              n408 = xnode "FPGA I/O Node"("I/O Item"=w925, "FPGA I/O In"=refnum<k21> "IO Socket\\SI 3 Deserializer MFP 5 Output") -> ()  [unwired: 1 out]
              n409 = xnode "FPGA I/O Node"("I/O Item"=w924, "FPGA I/O In"=refnum<k21> "IO Socket\\SI 3 Deserializer MFP 6 Output") -> ()  [unwired: 1 out]
              n410 = xnode "FPGA I/O Node"("I/O Item"=w916, "FPGA I/O In"=refnum<k21> "IO Socket\\SI 3 Deserializer MFP 7 Output") -> ()  [unwired: 1 out]
              n411 = xnode "FPGA I/O Node"("I/O Item"=w917, "FPGA I/O In"=refnum<k21> "IO Socket\\SI 3 Deserializer MFP 8 Output") -> ()  [unwired: 1 out]
              n412 = xnode "FPGA I/O Node"("I/O Item"=w918, "FPGA I/O In"=refnum<k21> "IO Socket\\SI 3 Deserializer MFP 9 Output") -> ()  [unwired: 1 out]
              n413 = xnode "FPGA I/O Node"("I/O Item"=w919, "FPGA I/O In"=refnum<k21> "IO Socket\\SI 3 Deserializer MFP 10 Output") -> ()  [unwired: 1 out]
            }
            frame "SO 0 Serializer" {
              n414 = xnode "FPGA I/O Node"("I/O Item"=w943, "FPGA I/O In"=refnum<k21> "IO Socket\\SO 0 Serializer MFP 0 Output") -> ()  [unwired: 1 out]
              n415 = xnode "FPGA I/O Node"("I/O Item"=w942, "FPGA I/O In"=refnum<k21> "IO Socket\\SO 0 Serializer MFP 3 Output") -> ()  [unwired: 1 out]
              n416 = xnode "FPGA I/O Node"("I/O Item"=w938, "FPGA I/O In"=refnum<k21> "IO Socket\\SO 0 Serializer MFP 4 Output") -> ()  [unwired: 1 out]
              n417 = xnode "FPGA I/O Node"("I/O Item"=w937, "FPGA I/O In"=refnum<k21> "IO Socket\\SO 0 Serializer MFP 6 Output") -> ()  [unwired: 1 out]
              n418 = xnode "FPGA I/O Node"("I/O Item"=w936, "FPGA I/O In"=refnum<k21> "IO Socket\\SO 0 Serializer MFP 7 Output") -> ()  [unwired: 1 out]
              n419 = xnode "FPGA I/O Node"("I/O Item"=w934, "FPGA I/O In"=refnum<k21> "IO Socket\\SO 0 Serializer MFP 8 Output") -> ()  [unwired: 1 out]
            }
            frame "SO 1 Serializer" {
              n420 = xnode "FPGA I/O Node"("I/O Item"=w955, "FPGA I/O In"=refnum<k21> "IO Socket\\SO 1 Serializer MFP 0 Output") -> ()  [unwired: 1 out]
              n421 = xnode "FPGA I/O Node"("I/O Item"=w954, "FPGA I/O In"=refnum<k21> "IO Socket\\SO 1 Serializer MFP 3 Output") -> ()  [unwired: 1 out]
              n422 = xnode "FPGA I/O Node"("I/O Item"=w950, "FPGA I/O In"=refnum<k21> "IO Socket\\SO 1 Serializer MFP 4 Output") -> ()  [unwired: 1 out]
              n423 = xnode "FPGA I/O Node"("I/O Item"=w949, "FPGA I/O In"=refnum<k21> "IO Socket\\SO 1 Serializer MFP 6 Output") -> ()  [unwired: 1 out]
              n424 = xnode "FPGA I/O Node"("I/O Item"=w948, "FPGA I/O In"=refnum<k21> "IO Socket\\SO 1 Serializer MFP 7 Output") -> ()  [unwired: 1 out]
              n425 = xnode "FPGA I/O Node"("I/O Item"=w946, "FPGA I/O In"=refnum<k21> "IO Socket\\SO 1 Serializer MFP 8 Output") -> ()  [unwired: 1 out]
            }
            frame "SO 2 Serializer" {
              n426 = xnode "FPGA I/O Node"("I/O Item"=w967, "FPGA I/O In"=refnum<k21> "IO Socket\\SO 2 Serializer MFP 0 Output") -> ()  [unwired: 1 out]
              n427 = xnode "FPGA I/O Node"("I/O Item"=w966, "FPGA I/O In"=refnum<k21> "IO Socket\\SO 2 Serializer MFP 3 Output") -> ()  [unwired: 1 out]
              n428 = xnode "FPGA I/O Node"("I/O Item"=w962, "FPGA I/O In"=refnum<k21> "IO Socket\\SO 2 Serializer MFP 4 Output") -> ()  [unwired: 1 out]
              n429 = xnode "FPGA I/O Node"("I/O Item"=w961, "FPGA I/O In"=refnum<k21> "IO Socket\\SO 2 Serializer MFP 6 Output") -> ()  [unwired: 1 out]
              n430 = xnode "FPGA I/O Node"("I/O Item"=w960, "FPGA I/O In"=refnum<k21> "IO Socket\\SO 2 Serializer MFP 7 Output") -> ()  [unwired: 1 out]
              n431 = xnode "FPGA I/O Node"("I/O Item"=w958, "FPGA I/O In"=refnum<k21> "IO Socket\\SO 2 Serializer MFP 8 Output") -> ()  [unwired: 1 out]
            }
            frame "SO 3 Serializer" {
              n432 = xnode "FPGA I/O Node"("I/O Item"=w979, "FPGA I/O In"=refnum<k21> "IO Socket\\SO 3 Serializer MFP 0 Output") -> ()  [unwired: 1 out]
              n433 = xnode "FPGA I/O Node"("I/O Item"=w978, "FPGA I/O In"=refnum<k21> "IO Socket\\SO 3 Serializer MFP 3 Output") -> ()  [unwired: 1 out]
              n434 = xnode "FPGA I/O Node"("I/O Item"=w974, "FPGA I/O In"=refnum<k21> "IO Socket\\SO 3 Serializer MFP 4 Output") -> ()  [unwired: 1 out]
              n435 = xnode "FPGA I/O Node"("I/O Item"=w973, "FPGA I/O In"=refnum<k21> "IO Socket\\SO 3 Serializer MFP 6 Output") -> ()  [unwired: 1 out]
              n436 = xnode "FPGA I/O Node"("I/O Item"=w972, "FPGA I/O In"=refnum<k21> "IO Socket\\SO 3 Serializer MFP 7 Output") -> ()  [unwired: 1 out]
              n437 = xnode "FPGA I/O Node"("I/O Item"=w970, "FPGA I/O In"=refnum<k21> "IO Socket\\SO 3 Serializer MFP 8 Output") -> ()  [unwired: 1 out]
            }
          }
          n438 = Not(x=w852) -> (.not. x?=w851:bool)
        }
        frame condition #11 {
          n439 = case shown="\"SO 0 Serializer\"" w995 {
            tunnel: w994 -> [_ w1009 w1027 w1042 w1054]
            tunnel: w993 -> [_ w1008 w1026 _ _]
            tunnel: w992 -> [_ _ _ _ _]
            tunnel: w991 -> [_ _ _ w1041 w1053]
            tunnel: w990 -> [_ w1007 w1025 w1037 w1049]
            tunnel: w989 -> [_ w1006 w1024 _ _]
            tunnel: w988 -> [_ w1005 w1023 w1036 w1048]
            tunnel: [w996 _ _ _ _] -> w987
            tunnel: w985 -> [_ w997 w1015 w1035 w1047]
            tunnel: w984 -> [_ w998 w1016 w1033 w1045]
            tunnel: w983 -> [_ w999 w1017 _ _]
            tunnel: w982 -> [_ w1000 w1018 _ _]
            frame Default {
              w996 = TRUE  # serdes id invalid
            }
            frame "SI 0 Deserializer" {
              n440 = xnode "FPGA I/O Node"("I/O Item"=w1009, "FPGA I/O In"=refnum<k21> "IO Socket\\SI 0 Deserializer MFP 0 Output") -> ()  [unwired: 1 out]
              n441 = xnode "FPGA I/O Node"("I/O Item"=w1008, "FPGA I/O In"=refnum<k21> "IO Socket\\SI 0 Deserializer MFP 1 Output") -> ()  [unwired: 1 out]
              n442 = xnode "FPGA I/O Node"("I/O Item"=w1007, "FPGA I/O In"=refnum<k21> "IO Socket\\SI 0 Deserializer MFP 4 Output") -> ()  [unwired: 1 out]
              n443 = xnode "FPGA I/O Node"("I/O Item"=w1006, "FPGA I/O In"=refnum<k21> "IO Socket\\SI 0 Deserializer MFP 5 Output") -> ()  [unwired: 1 out]
              n444 = xnode "FPGA I/O Node"("I/O Item"=w1005, "FPGA I/O In"=refnum<k21> "IO Socket\\SI 0 Deserializer MFP 6 Output") -> ()  [unwired: 1 out]
              n445 = xnode "FPGA I/O Node"("I/O Item"=w997, "FPGA I/O In"=refnum<k21> "IO Socket\\SI 0 Deserializer MFP 7 Output") -> ()  [unwired: 1 out]
              n446 = xnode "FPGA I/O Node"("I/O Item"=w998, "FPGA I/O In"=refnum<k21> "IO Socket\\SI 0 Deserializer MFP 8 Output") -> ()  [unwired: 1 out]
              n447 = xnode "FPGA I/O Node"("I/O Item"=w999, "FPGA I/O In"=refnum<k21> "IO Socket\\SI 0 Deserializer MFP 9 Output") -> ()  [unwired: 1 out]
              n448 = xnode "FPGA I/O Node"("I/O Item"=w1000, "FPGA I/O In"=refnum<k21> "IO Socket\\SI 0 Deserializer MFP 10 Output") -> ()  [unwired: 1 out]
            }
            frame "SI 1 Deserializer" {
              n449 = xnode "FPGA I/O Node"("I/O Item"=w1027, "FPGA I/O In"=refnum<k21> "IO Socket\\SI 1 Deserializer MFP 0 Output") -> ()  [unwired: 1 out]
              n450 = xnode "FPGA I/O Node"("I/O Item"=w1026, "FPGA I/O In"=refnum<k21> "IO Socket\\SI 1 Deserializer MFP 1 Output") -> ()  [unwired: 1 out]
              n451 = xnode "FPGA I/O Node"("I/O Item"=w1025, "FPGA I/O In"=refnum<k21> "IO Socket\\SI 1 Deserializer MFP 4 Output") -> ()  [unwired: 1 out]
              n452 = xnode "FPGA I/O Node"("I/O Item"=w1024, "FPGA I/O In"=refnum<k21> "IO Socket\\SI 1 Deserializer MFP 5 Output") -> ()  [unwired: 1 out]
              n453 = xnode "FPGA I/O Node"("I/O Item"=w1023, "FPGA I/O In"=refnum<k21> "IO Socket\\SI 1 Deserializer MFP 6 Output") -> ()  [unwired: 1 out]
              n454 = xnode "FPGA I/O Node"("I/O Item"=w1015, "FPGA I/O In"=refnum<k21> "IO Socket\\SI 1 Deserializer MFP 7 Output") -> ()  [unwired: 1 out]
              n455 = xnode "FPGA I/O Node"("I/O Item"=w1016, "FPGA I/O In"=refnum<k21> "IO Socket\\SI 1 Deserializer MFP 8 Output") -> ()  [unwired: 1 out]
              n456 = xnode "FPGA I/O Node"("I/O Item"=w1017, "FPGA I/O In"=refnum<k21> "IO Socket\\SI 1 Deserializer MFP 9 Output") -> ()  [unwired: 1 out]
              n457 = xnode "FPGA I/O Node"("I/O Item"=w1018, "FPGA I/O In"=refnum<k21> "IO Socket\\SI 1 Deserializer MFP 10 Output") -> ()  [unwired: 1 out]
            }
            frame "SO 0 Serializer" {
              n458 = xnode "FPGA I/O Node"("I/O Item"=w1042, "FPGA I/O In"=refnum<k21> "IO Socket\\SO 0 Serializer MFP 0 Output") -> ()  [unwired: 1 out]
              n459 = xnode "FPGA I/O Node"("I/O Item"=w1041, "FPGA I/O In"=refnum<k21> "IO Socket\\SO 0 Serializer MFP 3 Output") -> ()  [unwired: 1 out]
              n460 = xnode "FPGA I/O Node"("I/O Item"=w1037, "FPGA I/O In"=refnum<k21> "IO Socket\\SO 0 Serializer MFP 4 Output") -> ()  [unwired: 1 out]
              n461 = xnode "FPGA I/O Node"("I/O Item"=w1036, "FPGA I/O In"=refnum<k21> "IO Socket\\SO 0 Serializer MFP 6 Output") -> ()  [unwired: 1 out]
              n462 = xnode "FPGA I/O Node"("I/O Item"=w1035, "FPGA I/O In"=refnum<k21> "IO Socket\\SO 0 Serializer MFP 7 Output") -> ()  [unwired: 1 out]
              n463 = xnode "FPGA I/O Node"("I/O Item"=w1033, "FPGA I/O In"=refnum<k21> "IO Socket\\SO 0 Serializer MFP 8 Output") -> ()  [unwired: 1 out]
            }
            frame "SO 1 Serializer" {
              n464 = xnode "FPGA I/O Node"("I/O Item"=w1054, "FPGA I/O In"=refnum<k21> "IO Socket\\SO 1 Serializer MFP 0 Output") -> ()  [unwired: 1 out]
              n465 = xnode "FPGA I/O Node"("I/O Item"=w1053, "FPGA I/O In"=refnum<k21> "IO Socket\\SO 1 Serializer MFP 3 Output") -> ()  [unwired: 1 out]
              n466 = xnode "FPGA I/O Node"("I/O Item"=w1049, "FPGA I/O In"=refnum<k21> "IO Socket\\SO 1 Serializer MFP 4 Output") -> ()  [unwired: 1 out]
              n467 = xnode "FPGA I/O Node"("I/O Item"=w1048, "FPGA I/O In"=refnum<k21> "IO Socket\\SO 1 Serializer MFP 6 Output") -> ()  [unwired: 1 out]
              n468 = xnode "FPGA I/O Node"("I/O Item"=w1047, "FPGA I/O In"=refnum<k21> "IO Socket\\SO 1 Serializer MFP 7 Output") -> ()  [unwired: 1 out]
              n469 = xnode "FPGA I/O Node"("I/O Item"=w1045, "FPGA I/O In"=refnum<k21> "IO Socket\\SO 1 Serializer MFP 8 Output") -> ()  [unwired: 1 out]
            }
          }
          n470 = Not(x=w987) -> (.not. x?=w986:bool)
        }
      }
    }
  }
  "serdes id valid" <- w2
